vi "graph3.vi"(11 "replay":bool) -> (0 "path_size":i32, 3 "XY Graph":cluster{"Y":dbl[], "Y":dbl[]}[](graph)=[{"Y"=[-25.865695246715575, -25.865695246715575, -25.865695246715575], "Y"=[59.163033466791006, 59.163033466791006, 59.163033466791006]}, {"Y"=[0.85, 0.95, 0.95, 0.6, 0.6, 0.85, 0.85, -0.85, -0.85, -0.95, -0.95, -0.6, -0.6, -0.85, -0.6, -0.6, -0.85, -0.85, 0.85, 0.85], "Y"=[-0.6, -0.6, -1.4, -1.4, -0.6, -0.6, 2.4, 2.4, -0.6, -0.6, -1.4, -1.4, -0.6, -0.6, -0.6, -1.4, -1.4, -1.6, -1.6, -1.4]}, {"Y"=[-25.865695246715575], "Y"=[59.163033466791006]}, {"Y"=[], "Y"=[]}, {"Y"=array[926 elements], "Y"=array[926 elements]}, {"Y"=[nan, nan], "Y"=[nan, nan]}, {"Y"=[-25.865695246715575], "Y"=[59.163033466791006]}, {"Y"=[], "Y"=[]}, {"Y"=[], "Y"=[]}, {"Y"=[0.0], "Y"=[0.0]}, {"Y"=[], "Y"=[]}, {"Y"=[], "Y"=[]}, {"Y"=[691.7888277244315, 691.8377331659157, 691.8864790442867, 691.9350679862869, 691.9835025898547, 692.0317854247338, 692.079919033068, 692.1279059299806, 692.1757486041453, 692.2234495183519, 692.2710111100497, 692.3184357918904, 692.365725952261, 692.412883955801, 692.4599121439145, 692.5068128352747, 692.5535883263143, 692.6002408917145, 692.6467727848759, 692.6931862383941, 692.7394834645125, 692.785666655583, 692.8317379845035, 692.8776996051629, 692.9235536528688, 692.969302244769, 693.0149474802747, 693.060491441465, 693.1059361934975, 693.151283785001, 693.196536248471, 693.2416956006535, 693.2867638429291, 693.3317429616844, 693.3766349286853, 693.4214417014377, 693.4661652235502, 693.5108074250859, 693.5553702229134, 693.5998555210545, 693.6442652110193, 693.6886011721464, 693.7328652719325, 693.7770593663641, 693.8211853002351, 693.8652449074733, 693.9092400114525, 693.9531724253069, 693.9970439522381, 694.0408563858227, 694.0846115103164, 694.1283111009493, 694.1719569242241, 694.2155507382114, 694.259094292835, 694.3025893301664, 694.3460375847027, 694.3894407836557, 694.4328006472265, 694.476118888889, 694.5193972156585, 694.5626373283712, 694.6058409219545, 694.6490096856918, 694.6921453034947, 694.7352494541701, 694.7783238116778, 694.8213700453995, 694.8643898203949, 694.9073847976673, 694.9503566344149, 694.9933069842926, 695.0362374976652, 695.079149821865, 695.1220456014439, 695.1649264784243, 695.2077940925565, 695.2506500815632, 695.2934960813969, 695.3363337264864, 695.3791646499868, 695.4219904840265, 695.464812859962, 695.5076334086223, 695.5504537605557, 695.5932755462828, 695.6361003965429, 695.6789299425405, 695.7217658161954, 695.7646096503946, 695.807463079234, 695.8503277382761, 695.8932052647941, 695.9360972980251], "Y"=[-402.1714380892973, -402.2324443015287, -402.29325146963055, -402.3538628702814, -402.4142817442331, -402.47451129706894, -402.53455469993827, -402.5944150902866, -402.6540955725668, -402.71359921893855, -402.7729290699565, -402.832088135239, -402.8910793941361, -402.9499057963747, -403.00857026269705, -403.0670756854909, -403.12542492940014, -403.18362083193375, -403.24166620405737, -403.2995638307791, -403.3573164717253, -403.4149268617041, -403.4723977112591, -403.5297317072198, -403.58693151323575, -403.64399977030746, -403.7009390973042, -403.7577520914824, -403.81444132898264, -403.8710093653304, -403.9274587359257, -403.98379195652205, -404.0400115237071, -404.09611991536156, -404.1521195911291, -404.2080129928654, -404.2638025450895, -404.3194906554251, -404.375079715037, -404.4305720990579, -404.4859701670225, -404.5412762632748, -404.596492717394, -404.6516218445924, -404.70666594612766, -404.76162730969963, -404.81650820984265, -404.87131090831787, -404.9260376544974, -404.98069068574665, -405.0352722278018, -405.0897844951429, -405.14422969136206, -405.19861000952994, -405.2529276325616, -405.30718473357007, -405.3613834762236, -405.41552601510165, -405.46961449603776, -405.52365105647283, -405.5776378257941, -405.6315769256789, -405.685470470432, -405.7393205673213, -405.7931293169138, -405.84689881340205, -405.90063114494075, -405.9543283939694, -406.0079926375368, -406.0616259476311, -406.11523039149404, -406.1688080319476, -406.2223609277105, -406.2758911337184, -406.3294007014348, -406.38289167917463, -406.4363661124128, -406.4898260440976, -406.54327351496966, -406.5967105638653, -406.65013922803496, -406.70356154344927, -406.75697954511423, -406.8103952673769, -406.8638107442369, -406.9172280096572, -406.97064909787343, -407.0240760437018, -407.0775108828543, -407.1309556522436, -407.18441239029335, -407.23788313725817, -407.2913699355226, -407.3448748299264]}, {"Y"=[], "Y"=[]}, {"Y"=[-0.152017305614708], "Y"=[0.5451838106381299]}])   [LabVIEW 2015]
uses:
  G_NAV.vi
  G_VEH.vi
  G_SEN.vi
  G_PATH.vi
  <vilib>/Analysis/Matrix/Datatypes/RealMatrix.ctl
  <vilib>/Analysis/Matrix/NI_Matrix.lvlib
  <vilib>/Analysis/NI_AALBase.lvlib
  G_LCM.vi
  <vilib>/Analysis/baseanly.llb/Real A x B.vi
  G_ALL.vi
panel:
  out "x 17":dbl[](array[numeric])=[-13.0, -13.0, -13.0, -13.0, -13.0, -13.0, -13.0, -13.0, -13.0, -13.0, -13.0, -13.0, -13.0, -13.0, -13.0, -13.0, -13.0, -13.0, -13.0, -13.0, -13.0, -13.0, -13.0, -13.0, -13.0, -13.25, -13.25, -13.25, -13.25, -13.25, -13.25, -13.25, -13.25, -13.25, -13.25, -13.25, -13.25, -13.25, -13.25, -13.25, -13.25, -13.25, -13.25, -13.25, -13.25, -13.5, -13.25, -13.25, -13.25, -13.5, -13.5, -13.25, -13.5, -13.5, -13.5, -13.5, -13.5, -13.25, -13.5, -13.5, -13.75, -13.5, -13.5, -13.25, -13.75, -13.75, -13.5, -13.5, -13.5, -14.0, -14.0, -14.0, -13.75, -13.75, -13.75, -13.75, -1.0, -1.0, -0.75, -0.75, -0.75, -0.5, -0.5, -0.5, -0.25, -0.25, -0.25, -0.25, 0.0, 0.0, 0.0, 0.0, 0.0, 0.25, 0.25, 0.25, 0.25, 0.25, 0.5, 0.5, 0.5, 0.5, 0.75, 0.75, 0.75, 1.0, 1.0, 1.25, 1.25, 1.25, 1.5, 1.5]
  out "y 17":dbl[](array[numeric])=[0.0, 0.25, 0.5, 0.75, 1.0, 1.25, 1.25, 1.5, 1.75, 2.0, 2.25, 2.5, 2.75, 3.0, 3.25, 3.5, 3.75, 4.0, 4.25, 4.5, 4.75, 5.0, 5.25, 5.5, 5.75, 6.0, 6.5, 6.75, 7.0, 7.25, 7.5, 8.0, 8.25, 8.5, 9.0, 9.25, 9.5, 10.0, 10.25, 10.75, 11.25, 11.5, 12.0, 12.5, 13.0, 13.5, 13.75, 14.25, 14.75, 15.5, 16.0, 16.5, 17.25, 18.0, 18.5, 19.5, 20.0, 20.5, 21.75, 22.25, 23.75, 24.5, 25.25, 26.25, 28.25, 29.25, 30.5, 31.75, 33.25, 36.5, 38.25, 40.5, 42.75, 45.25, 48.25, 51.5, 4.25, 4.0, 4.0, 4.0, 3.75, 3.75, 3.75, 3.5, 3.5, 3.5, 3.25, 3.25, 3.25, 3.25, 3.25, 3.25, 3.0, 3.0, 3.0, 3.0, 3.0, 2.75, 3.0, 3.0, 3.0, 3.25, 3.25, 3.25, 3.5, 3.5, 3.5, 3.75, 3.75, 4.0, 4.0, 4.25]
  out "x 16":dbl[](array[numeric])=[-13.0, -13.0, -13.0, -13.0, -13.0, -13.0, -13.0, -13.0, -13.0, -13.0, -13.0, -13.0, -13.0, -13.0, -13.0, -13.0, -13.0, -13.0, -13.0, -13.0, -13.0, -13.0, -13.0, -13.0, -13.0, -13.25, -13.25, -13.25, -13.25, -13.25, -13.25, -13.25, -13.25, -13.25, -13.25, -13.25, -13.25, -13.25, -13.25, -13.25, -13.25, -13.25, -13.25, -13.25, -13.25, -13.5, -13.25, -13.25, -13.25, -13.5, -13.5, -13.25, -13.5, -13.5, -13.5, -13.5, -13.5, -13.25, -13.5, -13.5, -13.75, -13.5, -13.5, -13.25, -13.75, -13.75, -13.5, -13.5, -13.5, -14.0, -14.0, -14.0, -13.75, -13.75, -13.75, -13.75, -1.0, -1.0, -0.75, -0.75, -0.75, -0.5, -0.5, -0.5, -0.25, -0.25, -0.25, -0.25, 0.0, 0.0, 0.0, 0.0, 0.0, 0.25, 0.25, 0.25, 0.25, 0.25, 0.5, 0.5, 0.5, 0.5, 0.75, 0.75, 0.75, 1.0, 1.0, 1.25, 1.25, 1.25, 1.5, 1.5]
  out "y 16":dbl[](array[numeric])=[0.0, 0.25, 0.5, 0.75, 1.0, 1.25, 1.25, 1.5, 1.75, 2.0, 2.25, 2.5, 2.75, 3.0, 3.25, 3.5, 3.75, 4.0, 4.25, 4.5, 4.75, 5.0, 5.25, 5.5, 5.75, 6.0, 6.5, 6.75, 7.0, 7.25, 7.5, 8.0, 8.25, 8.5, 9.0, 9.25, 9.5, 10.0, 10.25, 10.75, 11.25, 11.5, 12.0, 12.5, 13.0, 13.5, 13.75, 14.25, 14.75, 15.5, 16.0, 16.5, 17.25, 18.0, 18.5, 19.5, 20.0, 20.5, 21.75, 22.25, 23.75, 24.5, 25.25, 26.25, 28.25, 29.25, 30.5, 31.75, 33.25, 36.5, 38.25, 40.5, 42.75, 45.25, 48.25, 51.5, 4.25, 4.0, 4.0, 4.0, 3.75, 3.75, 3.75, 3.5, 3.5, 3.5, 3.25, 3.25, 3.25, 3.25, 3.25, 3.25, 3.0, 3.0, 3.0, 3.0, 3.0, 2.75, 3.0, 3.0, 3.0, 3.25, 3.25, 3.25, 3.5, 3.5, 3.5, 3.75, 3.75, 4.0, 4.0, 4.25]
  out "M6006":T1={"GPSTime"=22892800.0, "attitude[2]"=-0.6123908, "lcc[0]"=-970.47205, "lcc[1]"=200.52362, "heading_GPS"=-0.6106907} {"GPSTime" format="%#_6f"}
  out "y 5":dbl[](array[numeric])
  out "x 5":dbl[](array[numeric])
  out "y 4":dbl[](array[numeric])
  out "x 4":dbl[](array[numeric])
  out "y 6":dbl[](array[numeric])
  out "x 6":dbl[](array[numeric])
  out "x 14":dbl[](array[numeric])
  out "y 14":dbl[](array[numeric])
  out "y 10":dbl[](array[numeric])
  out "x 10":dbl[](array[numeric])
  out "y 1":dbl[](array[numeric])
  out "x 1":dbl[](array[numeric])
  out "y 15":dbl[](array[numeric])=[0.0, 0.25, 0.5, 0.75, 1.0, 1.25, 1.25, 1.5, 1.75, 2.0, 2.25, 2.5, 2.75, 3.0, 3.25, 3.5, 3.75, 4.0, 4.25, 4.5, 4.75, 5.0, 5.25, 5.5, 5.75, 6.0, 6.5, 6.75, 7.0, 7.25, 7.5, 8.0, 8.25, 8.5, 9.0, 9.25, 9.5, 10.0, 10.25, 10.75, 11.25, 11.5, 12.0, 12.5, 13.0, 13.5, 13.75, 14.25, 14.75, 15.5, 16.0, 16.5, 17.25, 18.0, 18.5, 19.5, 20.0, 20.5, 21.75, 22.25, 23.75, 24.5, 25.25, 26.25, 28.25, 29.25, 30.5, 31.75, 33.25, 36.5, 38.25, 40.5, 42.75, 45.25, 48.25, 51.5, 4.25, 4.0, 4.0, 4.0, 3.75, 3.75, 3.75, 3.5, 3.5, 3.5, 3.25, 3.25, 3.25, 3.25, 3.25, 3.25, 3.0, 3.0, 3.0, 3.0, 3.0, 2.75, 3.0, 3.0, 3.0, 3.25, 3.25, 3.25, 3.5, 3.5, 3.5, 3.75, 3.75, 4.0, 4.0, 4.25]
  out "x 15":dbl[](array[numeric])=[-13.0, -13.0, -13.0, -13.0, -13.0, -13.0, -13.0, -13.0, -13.0, -13.0, -13.0, -13.0, -13.0, -13.0, -13.0, -13.0, -13.0, -13.0, -13.0, -13.0, -13.0, -13.0, -13.0, -13.0, -13.0, -13.25, -13.25, -13.25, -13.25, -13.25, -13.25, -13.25, -13.25, -13.25, -13.25, -13.25, -13.25, -13.25, -13.25, -13.25, -13.25, -13.25, -13.25, -13.25, -13.25, -13.5, -13.25, -13.25, -13.25, -13.5, -13.5, -13.25, -13.5, -13.5, -13.5, -13.5, -13.5, -13.25, -13.5, -13.5, -13.75, -13.5, -13.5, -13.25, -13.75, -13.75, -13.5, -13.5, -13.5, -14.0, -14.0, -14.0, -13.75, -13.75, -13.75, -13.75, -1.0, -1.0, -0.75, -0.75, -0.75, -0.5, -0.5, -0.5, -0.25, -0.25, -0.25, -0.25, 0.0, 0.0, 0.0, 0.0, 0.0, 0.25, 0.25, 0.25, 0.25, 0.25, 0.5, 0.5, 0.5, 0.5, 0.75, 0.75, 0.75, 1.0, 1.0, 1.25, 1.25, 1.25, 1.5, 1.5]
  out "y 13":dbl[](array[numeric])=[0.0, 0.25, 0.5, 0.75, 1.0, 1.25, 1.25, 1.5, 1.75, 2.0, 2.25, 2.5, 2.75, 3.0, 3.25, 3.5, 3.75, 4.0, 4.25, 4.5, 4.75, 5.0, 5.25, 5.5, 5.75, 6.0, 6.5, 6.75, 7.0, 7.25, 7.5, 8.0, 8.25, 8.5, 9.0, 9.25, 9.5, 10.0, 10.25, 10.75, 11.25, 11.5, 12.0, 12.5, 13.0, 13.5, 13.75, 14.25, 14.75, 15.5, 16.0, 16.5, 17.25, 18.0, 18.5, 19.5, 20.0, 20.5, 21.75, 22.25, 23.75, 24.5, 25.25, 26.25, 28.25, 29.25, 30.5, 31.75, 33.25, 36.5, 38.25, 40.5, 42.75, 45.25, 48.25, 51.5, 4.25, 4.0, 4.0, 4.0, 3.75, 3.75, 3.75, 3.5, 3.5, 3.5, 3.25, 3.25, 3.25, 3.25, 3.25, 3.25, 3.0, 3.0, 3.0, 3.0, 3.0, 2.75, 3.0, 3.0, 3.0, 3.25, 3.25, 3.25, 3.5, 3.5, 3.5, 3.75, 3.75, 4.0, 4.0, 4.25]
  out "x 13":dbl[](array[numeric])=[-13.0, -13.0, -13.0, -13.0, -13.0, -13.0, -13.0, -13.0, -13.0, -13.0, -13.0, -13.0, -13.0, -13.0, -13.0, -13.0, -13.0, -13.0, -13.0, -13.0, -13.0, -13.0, -13.0, -13.0, -13.0, -13.25, -13.25, -13.25, -13.25, -13.25, -13.25, -13.25, -13.25, -13.25, -13.25, -13.25, -13.25, -13.25, -13.25, -13.25, -13.25, -13.25, -13.25, -13.25, -13.25, -13.5, -13.25, -13.25, -13.25, -13.5, -13.5, -13.25, -13.5, -13.5, -13.5, -13.5, -13.5, -13.25, -13.5, -13.5, -13.75, -13.5, -13.5, -13.25, -13.75, -13.75, -13.5, -13.5, -13.5, -14.0, -14.0, -14.0, -13.75, -13.75, -13.75, -13.75, -1.0, -1.0, -0.75, -0.75, -0.75, -0.5, -0.5, -0.5, -0.25, -0.25, -0.25, -0.25, 0.0, 0.0, 0.0, 0.0, 0.0, 0.25, 0.25, 0.25, 0.25, 0.25, 0.5, 0.5, 0.5, 0.5, 0.75, 0.75, 0.75, 1.0, 1.0, 1.25, 1.25, 1.25, 1.5, 1.5]
  out "y 12":dbl[](array[numeric])=[0.0, 0.25, 0.5, 0.75, 1.0, 1.25, 1.25, 1.5, 1.75, 2.0, 2.25, 2.5, 2.75, 3.0, 3.25, 3.5, 3.75, 4.0, 4.25, 4.5, 4.75, 5.0, 5.25, 5.5, 5.75, 6.0, 6.5, 6.75, 7.0, 7.25, 7.5, 8.0, 8.25, 8.5, 9.0, 9.25, 9.5, 10.0, 10.25, 10.75, 11.25, 11.5, 12.0, 12.5, 13.0, 13.5, 13.75, 14.25, 14.75, 15.5, 16.0, 16.5, 17.25, 18.0, 18.5, 19.5, 20.0, 20.5, 21.75, 22.25, 23.75, 24.5, 25.25, 26.25, 28.25, 29.25, 30.5, 31.75, 33.25, 36.5, 38.25, 40.5, 42.75, 45.25, 48.25, 51.5, 4.25, 4.0, 4.0, 4.0, 3.75, 3.75, 3.75, 3.5, 3.5, 3.5, 3.25, 3.25, 3.25, 3.25, 3.25, 3.25, 3.0, 3.0, 3.0, 3.0, 3.0, 2.75, 3.0, 3.0, 3.0, 3.25, 3.25, 3.25, 3.5, 3.5, 3.5, 3.75, 3.75, 4.0, 4.0, 4.25]
  out "x 12":dbl[](array[numeric])=[-13.0, -13.0, -13.0, -13.0, -13.0, -13.0, -13.0, -13.0, -13.0, -13.0, -13.0, -13.0, -13.0, -13.0, -13.0, -13.0, -13.0, -13.0, -13.0, -13.0, -13.0, -13.0, -13.0, -13.0, -13.0, -13.25, -13.25, -13.25, -13.25, -13.25, -13.25, -13.25, -13.25, -13.25, -13.25, -13.25, -13.25, -13.25, -13.25, -13.25, -13.25, -13.25, -13.25, -13.25, -13.25, -13.5, -13.25, -13.25, -13.25, -13.5, -13.5, -13.25, -13.5, -13.5, -13.5, -13.5, -13.5, -13.25, -13.5, -13.5, -13.75, -13.5, -13.5, -13.25, -13.75, -13.75, -13.5, -13.5, -13.5, -14.0, -14.0, -14.0, -13.75, -13.75, -13.75, -13.75, -1.0, -1.0, -0.75, -0.75, -0.75, -0.5, -0.5, -0.5, -0.25, -0.25, -0.25, -0.25, 0.0, 0.0, 0.0, 0.0, 0.0, 0.25, 0.25, 0.25, 0.25, 0.25, 0.5, 0.5, 0.5, 0.5, 0.75, 0.75, 0.75, 1.0, 1.0, 1.25, 1.25, 1.25, 1.5, 1.5]
  out "y 11":dbl[](array[numeric])=[0.0, 0.25, 0.5, 0.75, 1.0, 1.25, 1.25, 1.5, 1.75, 2.0, 2.25, 2.5, 2.75, 3.0, 3.25, 3.5, 3.75, 4.0, 4.25, 4.5, 4.75, 5.0, 5.25, 5.5, 5.75, 6.0, 6.5, 6.75, 7.0, 7.25, 7.5, 8.0, 8.25, 8.5, 9.0, 9.25, 9.5, 10.0, 10.25, 10.75, 11.25, 11.5, 12.0, 12.5, 13.0, 13.5, 13.75, 14.25, 14.75, 15.5, 16.0, 16.5, 17.25, 18.0, 18.5, 19.5, 20.0, 20.5, 21.75, 22.25, 23.75, 24.5, 25.25, 26.25, 28.25, 29.25, 30.5, 31.75, 33.25, 36.5, 38.25, 40.5, 42.75, 45.25, 48.25, 51.5, 4.25, 4.0, 4.0, 4.0, 3.75, 3.75, 3.75, 3.5, 3.5, 3.5, 3.25, 3.25, 3.25, 3.25, 3.25, 3.25, 3.0, 3.0, 3.0, 3.0, 3.0, 2.75, 3.0, 3.0, 3.0, 3.25, 3.25, 3.25, 3.5, 3.5, 3.5, 3.75, 3.75, 4.0, 4.0, 4.25]
  out "x 11":dbl[](array[numeric])=[-13.0, -13.0, -13.0, -13.0, -13.0, -13.0, -13.0, -13.0, -13.0, -13.0, -13.0, -13.0, -13.0, -13.0, -13.0, -13.0, -13.0, -13.0, -13.0, -13.0, -13.0, -13.0, -13.0, -13.0, -13.0, -13.25, -13.25, -13.25, -13.25, -13.25, -13.25, -13.25, -13.25, -13.25, -13.25, -13.25, -13.25, -13.25, -13.25, -13.25, -13.25, -13.25, -13.25, -13.25, -13.25, -13.5, -13.25, -13.25, -13.25, -13.5, -13.5, -13.25, -13.5, -13.5, -13.5, -13.5, -13.5, -13.25, -13.5, -13.5, -13.75, -13.5, -13.5, -13.25, -13.75, -13.75, -13.5, -13.5, -13.5, -14.0, -14.0, -14.0, -13.75, -13.75, -13.75, -13.75, -1.0, -1.0, -0.75, -0.75, -0.75, -0.5, -0.5, -0.5, -0.25, -0.25, -0.25, -0.25, 0.0, 0.0, 0.0, 0.0, 0.0, 0.25, 0.25, 0.25, 0.25, 0.25, 0.5, 0.5, 0.5, 0.5, 0.75, 0.75, 0.75, 1.0, 1.0, 1.25, 1.25, 1.25, 1.5, 1.5]
  out "y 9":dbl[](array[numeric])=[-40.25486400827094, -40.04085960963455, -39.821235299880705, -39.59593792545196, -39.364914332790825, -39.12811136833988, -38.88547587854164, -38.636954709838655, -38.382494708673484, -38.12204272148863, -37.85554559472668, -37.58295017483014, -37.30420330824157, -37.0192518414035, -36.728042620758494, -36.43052249274907, -36.126638303817785, -35.81633690040717, -35.49956512895978, -35.176269835918156, -34.846397867724825, -34.50989607082233, -34.166711291653236, -33.81679037666006, -33.460080172285366, -33.09652752497168, -32.72607928116154, -32.3486822872975, -31.96428338982209, -31.57282943517787, -31.17426726980736, -30.768543740153135, -30.355605692657697, -30.338651341222633, -30.338651341222633, -29.95729378436619, -29.572397676750224, -29.183911226613308, -28.791782642194068, -28.395960131731087, -27.996391903462964, -27.593026165628288, -27.185811126465662, -26.774694994213668, -26.359625977110902, -25.940552283395995, -25.5174221213075, -25.090183699084033, -24.658785224964184, -24.22317490718656, -23.783300953989748, -23.33911157361234, -22.89055497429293, -22.43757936427013, -21.980132951782515, -21.5181639450687, -21.05162055236726, -20.58045098191681, -20.10460344195595, -19.62402614072324, -19.138667286457324, -18.648475087396758, -18.153397751780158, -17.653383487846114, -17.14838050383323, -16.6383370079801, -16.123201208525305, -15.602921313707439, -15.077445531765132, -14.546722070936944, -14.010699139461483, -13.469324945577348, -12.922547697523145, -12.370315603537431, -11.812576871858855, -11.249279710725965, -10.68037232837739, -10.105802933051706, -9.52551973298753, -8.939470936423437, -8.347604751598034, -8.312579060465806, -8.312579060465806, -7.815979397588906, -7.318560473773825, -6.820356240811432, -6.321400650492564, -5.8217276546080905, -5.321371204948849, -4.820365253305692, -4.318743751469474, -3.816540651231034, -3.313789904381253, -2.8105254627109564, -2.3067812780109964, -1.8025913020722415, -1.2979894866855162, -0.7930097836417018, -0.2876861447316371, 0.2179474782538381, 0.7238571335238572, 1.2300088692875666, 1.7363687337541345, 2.2429027751326935, 2.7495770416323975, 3.2563575814623866, 3.763210442831828, 4.270101673949855, 4.776997323025622, 5.283863438268267, 5.79066606788696, 6.297371260090832, 6.803945063089038, 7.310353525090725, 7.816562694305046, 8.322538618941149, 8.82824734720817, 9.333654927315276, 9.532792066869051, 9.532792066869058, 10.032676667529001, 10.532532309358876, 11.032359899557544, 11.53216034532386, 12.03193455385667, 12.53168343235485, 13.03140788801724, 13.531108828042706, 14.030787159630101, 14.530443789978285, 15.030079626286113, 15.529695575752449, 16.029292545576137, 16.52887144295605, 17.028433175091028, 17.527978649179936, 18.02750877242164, 18.527024452014977, 19.026526595158828, 19.526016109052026, 20.025493900893448, 20.52496087788194, 21.02441794721636, 21.523866016095567, 22.023305991718424, 22.522738781283774, 23.022165291990486, 23.521586431037413, 24.021003105623414, 24.520416222947343, 25.01982669020806, 25.51923541460442, 26.018643303335274, 26.518051263599492, 27.017460202595917, 27.51687102752342, 28.016284645580857, 28.515701963967068, 29.01512388988093, 29.51455133052128, 30.013985193087, 30.513426384776935, 31.012875812789932, 31.512334384324856, 32.01180300658057, 32.511282586755925, 33.01077403204978, 33.51027824966099, 34.00979614678842, 34.15163746485512, 34.15163746485511, 34.65085156194158, 35.150114036225105, 35.649423358614406, 36.148778000018126, 36.64817643134495, 37.14761712350358, 37.64709854740265, 38.14661917395086, 38.64617747405689, 39.14577191862942, 39.6454009785771, 40.14506312480863, 40.644756828232666, 41.14448055975791, 41.644232790293024, 42.14401199074667, 42.643816632027544, 43.14364518504432, 43.64349612070567, 44.14336790992027, 44.6432590235968, 45.14316793264393, 45.64309310797034, 46.143033020484694, 46.64298614109569, 47.14295094071199, 47.64292589024228, 48.14290946059522, 48.64290012267951, 49.142896347403784, 49.64289660567677, 50.142899368407114, 50.64290310650349, 51.14290629087459, 51.64290739242908, 52.14290488207564, 52.64289723072293, 53.142882909279656, 53.642860388654476, 54.14282813975608, 54.64278463349311, 55.14272834077427, 55.64265773250823, 56.14257127960367, 56.642467452969264, 57.142344723513695, 57.642201562145615, 58.14203643977374, 58.6418478273067, 59.141634195653204, 59.641394015721914, 60.1411257584215, 60.64082789466066, 61.14049889534806, 61.64013723139237, 62.139741373702265, 62.63930979318643, 63.138840960753534, 63.63833334731226, 64.13778542377129, 64.63719566103929, 65.1365625300249, 65.63588450163687, 66.13516004678382, 66.62661681170006, 66.62661681170006, 67.12576345342403, 67.62478981859165, 68.1236869902195, 68.62244605132406, 69.12105808492187, 69.61951417402948, 70.11780540166339, 70.61592285084015, 71.11385760457627, 71.61160074588827, 72.10914335779272, 72.6064765233061, 73.10359132544497, 73.60047884722584, 74.09713017166524, 74.59353638177971, 75.08968856058576, 75.58557779109994, 76.08119515633875, 76.57653173931875, 77.07157862305642, 77.56632689056836, 78.060767624871, 78.55489190898098, 79.04869082591473, 79.54215545868882, 80.03527689031979, 80.52804620382416, 81.02045448221844, 81.51249280851917, 82.00415226574289, 82.49542393690609, 82.98629890502534, 83.47676825311716, 83.96682306419804, 84.45645442128455, 84.9456534073932, 85.43441110554052, 85.92271859874306, 86.4105669700173, 86.89794730237979, 87.17622393756727, 87.17622393756727, 87.62090998324233, 88.06278904034333, 88.5018353078985, 88.93802298493607, 89.37132627048422, 89.80171936357122, 90.22917646322526, 90.65367176847454, 91.07517947834734, 91.49367379187183, 91.90912890807624, 92.3215190259888, 92.73081834463773, 93.13700106305124, 93.54004138025758, 93.93991349528491, 94.3365916071615, 94.73004991491554, 95.12026261757528, 95.50720391416891, 95.89084800372467, 96.27116908527078, 96.64814135783546, 97.02173902044692, 97.39193627213336, 97.75870731192305, 98.12202633884417, 98.48186755192496, 98.83820515019363, 99.19101333267841, 99.54026629840749, 99.88593824640913, 99.89953643323281, 99.89953643323281, 100.21054094201504, 100.51734678566943, 100.81989169992012, 101.11811342049135, 101.41194968310735, 101.70133822349231, 101.98621677737043, 102.26652308046596, 102.54219486850307, 102.81316987720602, 103.07938584229896, 103.34078049950615, 103.59729158455178, 103.84885683316006, 104.09541398105519, 104.33690076396141, 104.5732549176029, 104.80441417770389, 105.0303162799886, 105.2508989601812, 105.46609995400595, 105.67585699718703, 105.88010782544866, 106.07879017451506, 106.27184178011042, 106.45920037795898, 106.64080370378494, 106.81658949331246, 106.98649548226584, 107.15045940636924, 107.30841900134685, 107.46031200292295, 107.60607614682168, 107.74564916876727, 107.87896880448396, 108.00597278969595, 108.12659886012742, 108.24078475150262, 108.34846819954572, 108.44958693998096, 108.54407870853257, 108.63188124092471, 108.71293227288164, 108.78716954012754, 108.85453077838663, 108.91495372338314, 108.96837611084122, 108.97747618937277, 108.97747618937277, 109.0156550246946, 109.04983247580746, 109.08011123358501, 109.10659398890081, 109.12938343262847, 109.14858225564154, 109.16429314881364, 109.17661880301837, 109.18566190912927, 109.19152515801999, 109.19431124056405, 109.19412284763511, 109.1910626701067, 109.18523339885247, 109.17673772474595, 109.16567833866077, 109.15215793147051, 109.13627919404871, 109.11814481726906, 109.09785749200506, 109.07551990913035, 109.05123475951848, 109.02510473404305, 108.99723252357771, 108.96772081899594, 108.93667231117144, 108.90418969097772, 108.87037564928839, 108.83533287697705, 108.79916406491728, 108.7619719039827, 108.72385908504685, 108.68492829898334, 108.64528223666576, 108.60502358896771, 108.56425504676278, 108.52307930092454, 108.48159904232658, 108.4399169618425, 108.39813575034592, 108.35635809871036, 108.31468669780945, 108.27322423851678, 108.23207341170594, 108.19133690825049, 108.15111741902408, 108.11151763490025, 108.07264024675257, 108.03458794545469, 107.99746342188017, 107.96136936690259, 107.92640847139555, 107.89268342623265, 107.86029692228745, 107.82935165043357, 107.79995030154457, 107.78125898031978, 107.78125898031978, 107.75369240153198, 107.72548456275034, 107.69669916249154, 107.66739989927227, 107.63765047160923, 107.60751457801909, 107.57705591701853, 107.54633818712422, 107.51542508685286, 107.48438031472112, 107.45326756924571, 107.42215054894329, 107.39109295233057, 107.36015847792419, 107.32941082424084, 107.29891368979723, 107.26873077311004, 107.23892577269594, 107.2095623870716, 107.18070431475374, 107.15241525425903, 107.12475890410411, 107.09779896280573, 107.07159912888052, 107.04622310084521, 107.02173457721644, 106.9981972565109, 106.97567483724531, 106.95423101793631, 106.9339294971006, 106.91483397325487, 106.89700814491579, 106.88051571060006, 106.86545285263342, 106.86545285263342, 106.85123591176482, 106.8373215059327, 106.82369194296759, 106.81032953069995, 106.79721657696027, 106.78433538957903, 106.7716682763867, 106.75919754521381, 106.74690550389077, 106.73477446024813, 106.72278672211637, 106.71092459732593, 106.69917039370733, 106.68750641909104, 106.67591498130754, 106.66437838818732, 106.65287894756085, 106.64139896725864, 106.62992075511116, 106.61842661894889, 106.60689886660232, 106.59531980590192, 106.5836717446782, 106.57193699076163, 106.56009785198269, 106.54813663617186, 106.53603565115962, 106.52377720477648, 106.51134360485288, 106.49871715921937, 106.4858801757064, 106.47281496214443, 106.45950382636393, 106.44592907619545, 106.43207301946944, 106.41791796401637, 106.40344621766674, 106.38864008825105, 106.37348188359975, 106.35795391154335, 106.34203847991229, 106.32571789653713, 106.30897446924827, 106.29179050587625, 106.27414831425155, 106.2560637066309]
  out "x 9":dbl[](array[numeric])=[-22.968902627554595, -22.51700484334325, -22.067726202847595, -21.62109147813308, -21.177125441265126, -20.735852864309198, -20.297298519330727, -19.86148717839516, -19.42844361356793, -18.998192596914485, -18.57075890050028, -18.146167296390736, -17.724442556651315, -17.305609453347444, -16.889692758544577, -16.476717244308148, -16.0667076827036, -15.659688845796383, -15.255685505651932, -14.854722434335699, -14.456824403913117, -14.062016186449632, -13.67032255401068, -13.28176827866172, -12.896378132468183, -12.514176887495505, -12.135189315809143, -11.759440189474532, -11.38695428055711, -11.017756361122329, -10.651871203235629, -10.289323578962446, -9.930138260368233, -9.915595940630572, -9.915595940630572, -9.592217431479307, -9.27296664733781, -8.957904003376973, -8.64708991476769, -8.340584796680856, -8.038449064287356, -7.740743132758091, -7.447527417263952, -7.158862332975826, -6.874808295064605, -6.595425718701188, -6.320775019056462, -6.05091661130132, -5.7859109106066535, -5.525818332143363, -5.270699291082332, -5.02061420259445, -4.775623481850621, -4.535787544021732, -4.301166804278667, -4.071821677792334, -3.8478125797336116, -3.6291999252734, -3.4160441295825903, -3.2084056078320766, -3.0063447751927437, -2.809922046835485, -2.619197837931207, -2.4342325636507813, -2.255086639165114, -2.0818204796450988, -1.9144945002616136, -1.7531691161855663, -1.597904742587841, -1.4487617946393383, -1.3058006875109367, -1.1690818363735358, -1.0386656563980352, -0.9146125627553217, -0.796982970616279, -0.6858372951518088, -0.581235951532802, -0.4832393549301528, -0.3919079205147527, -0.30730206345748806, -0.22948219892925836, -0.22511372738602808, -0.22511372738602808, -0.16680067513880384, -0.11507613036628858, -0.06966705231019729, -0.03030040021222455, 0.0032968666859287954, 0.03139778914256819, 0.05427540791599236, 0.07220276376450722, 0.08545289744639678, 0.09429884971998208, 0.09901366134354672, 0.09987037307539658, 0.09714202567383796, 0.0911016598971616, 0.08202231650367428, 0.0701770362516814, 0.055838859899467026, 0.0392808282053517, 0.020775981927619973, 0.0005973618245841139, -0.020981991345463767, -0.043689036824225154, -0.06725073385338684, -0.09139404167465787, -0.11584591952973904, -0.14033332666033183, -0.164583222308123, -0.18832256571482164, -0.21127831612212852, -0.233177432771738, -0.25374687490535136, -0.27271360176467, -0.28980457259138814, -0.30474674662721396, -0.31726708311384183, -0.32147712013105156, -0.3214771201310518, -0.3322441522303675, -0.3444544578596952, -0.3580628233106866, -0.37302403487498664, -0.38929287884424707, -0.4068241415101202, -0.4255726091642576, -0.44549306809831846, -0.4665403046039335, -0.4886691049727688, -0.5118342554964762, -0.5359905424667011, -0.5610927521750875, -0.5870956709133022, -0.6139540849729826, -0.6416227806457879, -0.670056544223363, -0.6992101619973595, -0.72903842025943, -0.7594961053012258, -0.7905380034143993, -0.8221189008906022, -0.8541935840214723, -0.8867168390986828, -0.9196434524138646, -0.9529282102586762, -0.9865258989247632, -1.0203913047037911, -1.0544792138873982, -1.088744412767236, -1.1231416876349567, -1.1576258247822122, -1.192151610500654, -1.2266738310819347, -1.261147272817699, -1.2955267219995985, -1.329766964919293, -1.3638227878684193, -1.3976489771386371, -1.4312003190215978, -1.4644315998089543, -1.4972976057923506, -1.5297531232634387, -1.5617529385138709, -1.593251837835299, -1.6242046075193748, -1.6545660338577437, -1.684290903142064, -1.713334001663981, -1.7214502693093892, -1.721450269309389, -1.7494765704663608, -1.7766543195019637, -1.803010337186423, -1.8285714442899548, -1.8533644615827702, -1.8774162098350855, -1.9007535098171258, -1.9234031822991002, -1.9453920480512341, -1.966746927843737, -1.9874946424468334, -2.00766201263074, -2.027275859165667, -2.046363002821832, -2.0649502643694664, -2.083064464578773, -2.1007324242199688, -2.1179809640632783, -2.1348369048789184, -2.1513270674370997, -2.1674782725080464, -2.183317340861975, -2.198871093269103, -2.2141663504996414, -2.229229933323813, -2.244088662511829, -2.2587693588339204, -2.27329884306029, -2.2877039359611624, -2.3020114583067546, -2.316248230867277, -2.3304410744129536, -2.3446168097140014, -2.358802257540638, -2.3730242386630804, -2.387309573851546, -2.401685083876244, -2.4161775895074067, -2.430813911515237, -2.445620870669959, -2.46062528774179, -2.4758539835009468, -2.491333778717647, -2.5070914941621076, -2.523153950604546, -2.539547968815179, -2.556300369564224, -2.573437973621899, -2.5909876017584192, -2.6089760747440036, -2.6274302133488687, -2.646376838343232, -2.66584277049731, -2.68585483058132, -2.7064398393654807, -2.7276246176200143, -2.749435986115125, -2.7719007656210435, -2.7950457769079735, -2.818897840746146, -2.843483777905771, -2.8688304091570727, -2.8949645552702545, -2.921913037015548, -2.9492635082994942, -2.9492635082994942, -2.978480917327609, -3.0098270674333767, -3.043459777809386, -3.079536867648219, -3.118216156142463, -3.1596554624846984, -3.204012605867507, -3.2514454054834765, -3.3021116805251873, -3.3561692501852223, -3.4137759336561606, -3.4750895501305976, -3.5402679188011072, -3.6094688588602786, -3.682850189500691, -3.760569729914927, -3.842785299295573, -3.929654716835212, -4.021335801726423, -4.117986373161795, -4.219764250333915, -4.326827252435352, -4.439333198658707, -4.557439908196553, -4.6813052002414715, -4.811086893986051, -4.946942808622881, -5.089030763344532, -5.237508577343594, -5.392534069812648, -5.554265059944274, -5.722859366931069, -5.898474809965605, -6.081269208240471, -6.27140038094824, -6.469026147281509, -6.674304326432857, -6.88739273759486, -7.10844919996011, -7.33763153272119, -7.5750975550706805, -7.714565866361133, -7.714565866361133, -7.943178762901428, -8.177335605648189, -8.417087352842183, -8.6624849627242, -8.913579393535008, -9.170421603515402, -9.433062550906158, -9.701553193948051, -9.975944490881862, -10.256287399948372, -10.542632879388364, -10.835031887442614, -11.133535382351901, -11.438194322357017, -11.74905966569872, -12.06618237061781, -12.389613395355056, -12.719403698151243, -13.055604237247149, -13.398265970883559, -13.747439857301249, -14.10317685474099, -14.465527921443577, -14.83454401564979, -15.210276095600387, -15.592775119536174, -15.982092045697918, -16.378277832326408, -16.78138343766241, -17.19145981994672, -17.608557937420102, -18.032728748323343, -18.0496518526286, -18.0496518526286, -18.441165968034287, -18.83605201755941, -19.234360005438532, -19.636139935906236, -20.041441813197096, -20.450315641545686, -20.862811425186578, -21.278979168354343, -21.698868875283566, -22.122530550208822, -22.550014197364675, -22.98136982098571, -23.41664742530649, -23.8558970145616, -24.29916859298561, -24.746512164813097, -25.197977734278638, -25.6536153056168, -26.113474883062164, -26.5776064708493, -27.046060073212793, -27.5188856943872, -27.996133338607113, -28.4778530101071, -28.96409471312173, -29.454908451885586, -29.950344230633245, -30.450452053599268, -30.95528192501824, -31.46488384912474, -31.979307830153324, -32.49860387233859, -33.0228219799151, -33.552012157117424, -34.08622440818015, -34.625508737337846, -35.16991514882508, -35.719493646876444, -36.2742942357265, -36.83436691960981, -37.39976170276098, -37.97052858941455, -38.54671758380513, -39.12837869016727, -39.71556191273555, -40.308317255744555, -40.90669472342885, -41.01788165020217, -41.01788165020217, -41.516426075908484, -42.01529336894664, -42.514475243301945, -43.01396341295969, -43.51374959190518, -44.013825494123736, -44.514182833600636, -45.01481332432121, -45.515708680270734, -46.01686061543453, -46.51826084379791, -47.019901079346155, -47.521773036064594, -48.0238684279385, -48.526178968953204, -49.02869637309399, -49.53141235434619, -50.03431862669508, -50.53740690412599, -51.04066890062418, -51.54409633017501, -52.04768090676373, -52.55141434437569, -53.055288356996165, -53.55929465861046, -54.0634249632039, -54.56767098476177, -55.072024437269384, -55.576477034712035, -56.08102049107504, -56.58564652034369, -57.090346836503294, -57.59511315353915, -58.09993718543659, -58.60481064618088, -59.109725249757346, -59.61467271015128, -60.119644741348004, -60.62463305733281, -61.129629372090996, -61.63462539960787, -62.13961285386874, -62.64458344885892, -63.149528898563695, -63.65444091696837, -64.15931121805825, -64.66413151581865, -65.16889352423487, -65.67358895729222, -66.17820952897598, -66.68274695327148, -67.18719294416401, -67.69153921563887, -68.19577748168139, -68.69989945627682, -69.20389685341053, -69.53980106644636, -69.53980106644636, -70.03904068922449, -70.53824534388608, -71.03741850393202, -71.53656364286319, -72.03568423418045, -72.53478375138471, -73.03386566797683, -73.53293345745773, -74.03199059332825, -74.5310405490893, -75.03008679824175, -75.52913281428651, -76.02818207072443, -76.5272380410564, -77.02630419878331, -77.52538401740605, -78.02448097042549, -78.52359853134253, -79.02274017365804, -79.52190937087288, -80.02110959648799, -80.5203443240042, -81.01961702692243, -81.51893117874353, -82.01829025296841, -82.51769772309794, -83.01715706263303, -83.51667174507452, -84.01624524392331, -84.5158810326803, -85.01558258484634, -85.51535337392235, -86.0151968734092, -86.51398695208124, -86.51398695208124, -87.01378481453521, -87.51359137792667, -88.01340613342705, -88.51322857220782, -89.01305818544041, -89.51289446429632, -90.01273689994701, -90.51258498356393, -91.01243820631852, -91.5122960593823, -92.01215803392664, -92.51202362112309, -93.01189231214308, -93.51176359815807, -94.01163697033948, -94.51151191985885, -95.01138793788758, -95.51126451559716, -96.01114114415904, -96.51101731474469, -97.01089251852558, -97.51076624667314, -98.01063799035886, -98.5105072407542, -99.01037348903058, -99.51023622635952, -100.01009494391245, -100.50994913286084, -101.00979828437613, -101.50964188962982, -102.00947943979334, -102.50931042603817, -103.00913433953575, -103.50895067145754, -104.00875891297504, -104.50855855525968, -105.00834908948293, -105.50813000681626, -106.0079007984311, -106.50766095549893, -107.00740996919122, -107.50714733067944, -108.00687253113502, -108.50658506172944, -109.00628441363415, -109.50505830995377]
  out "x 7":dbl[](array[numeric])=[0.0, -0.062285707493046516, -0.2310475110116812]
  out "y 7":dbl[](array[numeric])=[0.0, 3.113870125529085, 5.994064450521981]
  out "y 8":dbl[](array[numeric])=[-40.25486400827094, -40.04085960963455, -39.821235299880705, -39.59593792545196, -39.364914332790825, -39.12811136833988, -38.88547587854164, -38.636954709838655, -38.382494708673484, -38.12204272148863, -37.85554559472668, -37.58295017483014, -37.30420330824157, -37.0192518414035, -36.728042620758494, -36.43052249274907, -36.126638303817785, -35.81633690040717, -35.49956512895978, -35.176269835918156, -34.846397867724825, -34.50989607082233, -34.166711291653236, -33.81679037666006, -33.460080172285366, -33.09652752497168, -32.72607928116154, -32.3486822872975, -31.96428338982209, -31.57282943517787, -31.17426726980736, -30.768543740153135, -30.355605692657697, -30.338651341222633, -30.338651341222633, -29.95729378436619, -29.572397676750224, -29.183911226613308, -28.791782642194068, -28.395960131731087, -27.996391903462964, -27.593026165628288, -27.185811126465662, -26.774694994213668, -26.359625977110902, -25.940552283395995, -25.5174221213075, -25.090183699084033, -24.658785224964184, -24.22317490718656, -23.783300953989748, -23.33911157361234, -22.89055497429293, -22.43757936427013, -21.980132951782515, -21.5181639450687, -21.05162055236726, -20.58045098191681, -20.10460344195595, -19.62402614072324, -19.138667286457324, -18.648475087396758, -18.153397751780158, -17.653383487846114, -17.14838050383323, -16.6383370079801, -16.123201208525305, -15.602921313707439, -15.077445531765132, -14.546722070936944, -14.010699139461483, -13.469324945577348, -12.922547697523145, -12.370315603537431, -11.812576871858855, -11.249279710725965, -10.68037232837739, -10.105802933051706, -9.52551973298753, -8.939470936423437, -8.347604751598034, -8.312579060465806, -8.312579060465806, -7.815979397588906, -7.318560473773825, -6.820356240811432, -6.321400650492564, -5.8217276546080905, -5.321371204948849, -4.820365253305692, -4.318743751469474, -3.816540651231034, -3.313789904381253, -2.8105254627109564, -2.3067812780109964, -1.8025913020722415, -1.2979894866855162, -0.7930097836417018, -0.2876861447316371, 0.2179474782538381, 0.7238571335238572, 1.2300088692875666, 1.7363687337541345, 2.2429027751326935, 2.7495770416323975, 3.2563575814623866, 3.763210442831828, 4.270101673949855, 4.776997323025622, 5.283863438268267, 5.79066606788696, 6.297371260090832, 6.803945063089038, 7.310353525090725, 7.816562694305046, 8.322538618941149, 8.82824734720817, 9.333654927315276, 9.532792066869051, 9.532792066869058, 10.032676667529001, 10.532532309358876, 11.032359899557544, 11.53216034532386, 12.03193455385667, 12.53168343235485, 13.03140788801724, 13.531108828042706, 14.030787159630101, 14.530443789978285, 15.030079626286113, 15.529695575752449, 16.029292545576137, 16.52887144295605, 17.028433175091028, 17.527978649179936, 18.02750877242164, 18.527024452014977, 19.026526595158828, 19.526016109052026, 20.025493900893448, 20.52496087788194, 21.02441794721636, 21.523866016095567, 22.023305991718424, 22.522738781283774, 23.022165291990486, 23.521586431037413, 24.021003105623414, 24.520416222947343, 25.01982669020806, 25.51923541460442, 26.018643303335274, 26.518051263599492, 27.017460202595917, 27.51687102752342, 28.016284645580857, 28.515701963967068, 29.01512388988093, 29.51455133052128, 30.013985193087, 30.513426384776935, 31.012875812789932, 31.512334384324856, 32.01180300658057, 32.511282586755925, 33.01077403204978, 33.51027824966099, 34.00979614678842, 34.15163746485512, 34.15163746485511, 34.65085156194158, 35.150114036225105, 35.649423358614406, 36.148778000018126, 36.64817643134495, 37.14761712350358, 37.64709854740265, 38.14661917395086, 38.64617747405689, 39.14577191862942, 39.6454009785771, 40.14506312480863, 40.644756828232666, 41.14448055975791, 41.644232790293024, 42.14401199074667, 42.643816632027544, 43.14364518504432, 43.64349612070567, 44.14336790992027, 44.6432590235968, 45.14316793264393, 45.64309310797034, 46.143033020484694, 46.64298614109569, 47.14295094071199, 47.64292589024228, 48.14290946059522, 48.64290012267951, 49.142896347403784, 49.64289660567677, 50.142899368407114, 50.64290310650349, 51.14290629087459, 51.64290739242908, 52.14290488207564, 52.64289723072293, 53.142882909279656, 53.642860388654476, 54.14282813975608, 54.64278463349311, 55.14272834077427, 55.64265773250823, 56.14257127960367, 56.642467452969264, 57.142344723513695, 57.642201562145615, 58.14203643977374, 58.6418478273067, 59.141634195653204, 59.641394015721914, 60.1411257584215, 60.64082789466066, 61.14049889534806, 61.64013723139237, 62.139741373702265, 62.63930979318643, 63.138840960753534, 63.63833334731226, 64.13778542377129, 64.63719566103929, 65.1365625300249, 65.63588450163687, 66.13516004678382, 66.62661681170006, 66.62661681170006, 67.12576345342403, 67.62478981859165, 68.1236869902195, 68.62244605132406, 69.12105808492187, 69.61951417402948, 70.11780540166339, 70.61592285084015, 71.11385760457627, 71.61160074588827, 72.10914335779272, 72.6064765233061, 73.10359132544497, 73.60047884722584, 74.09713017166524, 74.59353638177971, 75.08968856058576, 75.58557779109994, 76.08119515633875, 76.57653173931875, 77.07157862305642, 77.56632689056836, 78.060767624871, 78.55489190898098, 79.04869082591473, 79.54215545868882, 80.03527689031979, 80.52804620382416, 81.02045448221844, 81.51249280851917, 82.00415226574289, 82.49542393690609, 82.98629890502534, 83.47676825311716, 83.96682306419804, 84.45645442128455, 84.9456534073932, 85.43441110554052, 85.92271859874306, 86.4105669700173, 86.89794730237979, 87.17622393756727, 87.17622393756727, 87.62090998324233, 88.06278904034333, 88.5018353078985, 88.93802298493607, 89.37132627048422, 89.80171936357122, 90.22917646322526, 90.65367176847454, 91.07517947834734, 91.49367379187183, 91.90912890807624, 92.3215190259888, 92.73081834463773, 93.13700106305124, 93.54004138025758, 93.93991349528491, 94.3365916071615, 94.73004991491554, 95.12026261757528, 95.50720391416891, 95.89084800372467, 96.27116908527078, 96.64814135783546, 97.02173902044692, 97.39193627213336, 97.75870731192305, 98.12202633884417, 98.48186755192496, 98.83820515019363, 99.19101333267841, 99.54026629840749, 99.88593824640913, 99.89953643323281, 99.89953643323281, 100.21054094201504, 100.51734678566943, 100.81989169992012, 101.11811342049135, 101.41194968310735, 101.70133822349231, 101.98621677737043, 102.26652308046596, 102.54219486850307, 102.81316987720602, 103.07938584229896, 103.34078049950615, 103.59729158455178, 103.84885683316006, 104.09541398105519, 104.33690076396141, 104.5732549176029, 104.80441417770389, 105.0303162799886, 105.2508989601812, 105.46609995400595, 105.67585699718703, 105.88010782544866, 106.07879017451506, 106.27184178011042, 106.45920037795898, 106.64080370378494, 106.81658949331246, 106.98649548226584, 107.15045940636924, 107.30841900134685, 107.46031200292295, 107.60607614682168, 107.74564916876727, 107.87896880448396, 108.00597278969595, 108.12659886012742, 108.24078475150262, 108.34846819954572, 108.44958693998096, 108.54407870853257, 108.63188124092471, 108.71293227288164, 108.78716954012754, 108.85453077838663, 108.91495372338314, 108.96837611084122, 108.97747618937277, 108.97747618937277, 109.0156550246946, 109.04983247580746, 109.08011123358501, 109.10659398890081, 109.12938343262847, 109.14858225564154, 109.16429314881364, 109.17661880301837, 109.18566190912927, 109.19152515801999, 109.19431124056405, 109.19412284763511, 109.1910626701067, 109.18523339885247, 109.17673772474595, 109.16567833866077, 109.15215793147051, 109.13627919404871, 109.11814481726906, 109.09785749200506, 109.07551990913035, 109.05123475951848, 109.02510473404305, 108.99723252357771, 108.96772081899594, 108.93667231117144, 108.90418969097772, 108.87037564928839, 108.83533287697705, 108.79916406491728, 108.7619719039827, 108.72385908504685, 108.68492829898334, 108.64528223666576, 108.60502358896771, 108.56425504676278, 108.52307930092454, 108.48159904232658, 108.4399169618425, 108.39813575034592, 108.35635809871036, 108.31468669780945, 108.27322423851678, 108.23207341170594, 108.19133690825049, 108.15111741902408, 108.11151763490025, 108.07264024675257, 108.03458794545469, 107.99746342188017, 107.96136936690259, 107.92640847139555, 107.89268342623265, 107.86029692228745, 107.82935165043357, 107.79995030154457, 107.78125898031978, 107.78125898031978, 107.75369240153198, 107.72548456275034, 107.69669916249154, 107.66739989927227, 107.63765047160923, 107.60751457801909, 107.57705591701853, 107.54633818712422, 107.51542508685286, 107.48438031472112, 107.45326756924571, 107.42215054894329, 107.39109295233057, 107.36015847792419, 107.32941082424084, 107.29891368979723, 107.26873077311004, 107.23892577269594, 107.2095623870716, 107.18070431475374, 107.15241525425903, 107.12475890410411, 107.09779896280573, 107.07159912888052, 107.04622310084521, 107.02173457721644, 106.9981972565109, 106.97567483724531, 106.95423101793631, 106.9339294971006, 106.91483397325487, 106.89700814491579, 106.88051571060006, 106.86545285263342, 106.86545285263342, 106.85123591176482, 106.8373215059327, 106.82369194296759, 106.81032953069995, 106.79721657696027, 106.78433538957903, 106.7716682763867, 106.75919754521381, 106.74690550389077, 106.73477446024813, 106.72278672211637, 106.71092459732593, 106.69917039370733, 106.68750641909104, 106.67591498130754, 106.66437838818732, 106.65287894756085, 106.64139896725864, 106.62992075511116, 106.61842661894889, 106.60689886660232, 106.59531980590192, 106.5836717446782, 106.57193699076163, 106.56009785198269, 106.54813663617186, 106.53603565115962, 106.52377720477648, 106.51134360485288, 106.49871715921937, 106.4858801757064, 106.47281496214443, 106.45950382636393, 106.44592907619545, 106.43207301946944, 106.41791796401637, 106.40344621766674, 106.38864008825105, 106.37348188359975, 106.35795391154335, 106.34203847991229, 106.32571789653713, 106.30897446924827, 106.29179050587625, 106.27414831425155, 106.2560637066309]
  out "x 8":dbl[](array[numeric])=[-22.968902627554595, -22.51700484334325, -22.067726202847595, -21.62109147813308, -21.177125441265126, -20.735852864309198, -20.297298519330727, -19.86148717839516, -19.42844361356793, -18.998192596914485, -18.57075890050028, -18.146167296390736, -17.724442556651315, -17.305609453347444, -16.889692758544577, -16.476717244308148, -16.0667076827036, -15.659688845796383, -15.255685505651932, -14.854722434335699, -14.456824403913117, -14.062016186449632, -13.67032255401068, -13.28176827866172, -12.896378132468183, -12.514176887495505, -12.135189315809143, -11.759440189474532, -11.38695428055711, -11.017756361122329, -10.651871203235629, -10.289323578962446, -9.930138260368233, -9.915595940630572, -9.915595940630572, -9.592217431479307, -9.27296664733781, -8.957904003376973, -8.64708991476769, -8.340584796680856, -8.038449064287356, -7.740743132758091, -7.447527417263952, -7.158862332975826, -6.874808295064605, -6.595425718701188, -6.320775019056462, -6.05091661130132, -5.7859109106066535, -5.525818332143363, -5.270699291082332, -5.02061420259445, -4.775623481850621, -4.535787544021732, -4.301166804278667, -4.071821677792334, -3.8478125797336116, -3.6291999252734, -3.4160441295825903, -3.2084056078320766, -3.0063447751927437, -2.809922046835485, -2.619197837931207, -2.4342325636507813, -2.255086639165114, -2.0818204796450988, -1.9144945002616136, -1.7531691161855663, -1.597904742587841, -1.4487617946393383, -1.3058006875109367, -1.1690818363735358, -1.0386656563980352, -0.9146125627553217, -0.796982970616279, -0.6858372951518088, -0.581235951532802, -0.4832393549301528, -0.3919079205147527, -0.30730206345748806, -0.22948219892925836, -0.22511372738602808, -0.22511372738602808, -0.16680067513880384, -0.11507613036628858, -0.06966705231019729, -0.03030040021222455, 0.0032968666859287954, 0.03139778914256819, 0.05427540791599236, 0.07220276376450722, 0.08545289744639678, 0.09429884971998208, 0.09901366134354672, 0.09987037307539658, 0.09714202567383796, 0.0911016598971616, 0.08202231650367428, 0.0701770362516814, 0.055838859899467026, 0.0392808282053517, 0.020775981927619973, 0.0005973618245841139, -0.020981991345463767, -0.043689036824225154, -0.06725073385338684, -0.09139404167465787, -0.11584591952973904, -0.14033332666033183, -0.164583222308123, -0.18832256571482164, -0.21127831612212852, -0.233177432771738, -0.25374687490535136, -0.27271360176467, -0.28980457259138814, -0.30474674662721396, -0.31726708311384183, -0.32147712013105156, -0.3214771201310518, -0.3322441522303675, -0.3444544578596952, -0.3580628233106866, -0.37302403487498664, -0.38929287884424707, -0.4068241415101202, -0.4255726091642576, -0.44549306809831846, -0.4665403046039335, -0.4886691049727688, -0.5118342554964762, -0.5359905424667011, -0.5610927521750875, -0.5870956709133022, -0.6139540849729826, -0.6416227806457879, -0.670056544223363, -0.6992101619973595, -0.72903842025943, -0.7594961053012258, -0.7905380034143993, -0.8221189008906022, -0.8541935840214723, -0.8867168390986828, -0.9196434524138646, -0.9529282102586762, -0.9865258989247632, -1.0203913047037911, -1.0544792138873982, -1.088744412767236, -1.1231416876349567, -1.1576258247822122, -1.192151610500654, -1.2266738310819347, -1.261147272817699, -1.2955267219995985, -1.329766964919293, -1.3638227878684193, -1.3976489771386371, -1.4312003190215978, -1.4644315998089543, -1.4972976057923506, -1.5297531232634387, -1.5617529385138709, -1.593251837835299, -1.6242046075193748, -1.6545660338577437, -1.684290903142064, -1.713334001663981, -1.7214502693093892, -1.721450269309389, -1.7494765704663608, -1.7766543195019637, -1.803010337186423, -1.8285714442899548, -1.8533644615827702, -1.8774162098350855, -1.9007535098171258, -1.9234031822991002, -1.9453920480512341, -1.966746927843737, -1.9874946424468334, -2.00766201263074, -2.027275859165667, -2.046363002821832, -2.0649502643694664, -2.083064464578773, -2.1007324242199688, -2.1179809640632783, -2.1348369048789184, -2.1513270674370997, -2.1674782725080464, -2.183317340861975, -2.198871093269103, -2.2141663504996414, -2.229229933323813, -2.244088662511829, -2.2587693588339204, -2.27329884306029, -2.2877039359611624, -2.3020114583067546, -2.316248230867277, -2.3304410744129536, -2.3446168097140014, -2.358802257540638, -2.3730242386630804, -2.387309573851546, -2.401685083876244, -2.4161775895074067, -2.430813911515237, -2.445620870669959, -2.46062528774179, -2.4758539835009468, -2.491333778717647, -2.5070914941621076, -2.523153950604546, -2.539547968815179, -2.556300369564224, -2.573437973621899, -2.5909876017584192, -2.6089760747440036, -2.6274302133488687, -2.646376838343232, -2.66584277049731, -2.68585483058132, -2.7064398393654807, -2.7276246176200143, -2.749435986115125, -2.7719007656210435, -2.7950457769079735, -2.818897840746146, -2.843483777905771, -2.8688304091570727, -2.8949645552702545, -2.921913037015548, -2.9492635082994942, -2.9492635082994942, -2.978480917327609, -3.0098270674333767, -3.043459777809386, -3.079536867648219, -3.118216156142463, -3.1596554624846984, -3.204012605867507, -3.2514454054834765, -3.3021116805251873, -3.3561692501852223, -3.4137759336561606, -3.4750895501305976, -3.5402679188011072, -3.6094688588602786, -3.682850189500691, -3.760569729914927, -3.842785299295573, -3.929654716835212, -4.021335801726423, -4.117986373161795, -4.219764250333915, -4.326827252435352, -4.439333198658707, -4.557439908196553, -4.6813052002414715, -4.811086893986051, -4.946942808622881, -5.089030763344532, -5.237508577343594, -5.392534069812648, -5.554265059944274, -5.722859366931069, -5.898474809965605, -6.081269208240471, -6.27140038094824, -6.469026147281509, -6.674304326432857, -6.88739273759486, -7.10844919996011, -7.33763153272119, -7.5750975550706805, -7.714565866361133, -7.714565866361133, -7.943178762901428, -8.177335605648189, -8.417087352842183, -8.6624849627242, -8.913579393535008, -9.170421603515402, -9.433062550906158, -9.701553193948051, -9.975944490881862, -10.256287399948372, -10.542632879388364, -10.835031887442614, -11.133535382351901, -11.438194322357017, -11.74905966569872, -12.06618237061781, -12.389613395355056, -12.719403698151243, -13.055604237247149, -13.398265970883559, -13.747439857301249, -14.10317685474099, -14.465527921443577, -14.83454401564979, -15.210276095600387, -15.592775119536174, -15.982092045697918, -16.378277832326408, -16.78138343766241, -17.19145981994672, -17.608557937420102, -18.032728748323343, -18.0496518526286, -18.0496518526286, -18.441165968034287, -18.83605201755941, -19.234360005438532, -19.636139935906236, -20.041441813197096, -20.450315641545686, -20.862811425186578, -21.278979168354343, -21.698868875283566, -22.122530550208822, -22.550014197364675, -22.98136982098571, -23.41664742530649, -23.8558970145616, -24.29916859298561, -24.746512164813097, -25.197977734278638, -25.6536153056168, -26.113474883062164, -26.5776064708493, -27.046060073212793, -27.5188856943872, -27.996133338607113, -28.4778530101071, -28.96409471312173, -29.454908451885586, -29.950344230633245, -30.450452053599268, -30.95528192501824, -31.46488384912474, -31.979307830153324, -32.49860387233859, -33.0228219799151, -33.552012157117424, -34.08622440818015, -34.625508737337846, -35.16991514882508, -35.719493646876444, -36.2742942357265, -36.83436691960981, -37.39976170276098, -37.97052858941455, -38.54671758380513, -39.12837869016727, -39.71556191273555, -40.308317255744555, -40.90669472342885, -41.01788165020217, -41.01788165020217, -41.516426075908484, -42.01529336894664, -42.514475243301945, -43.01396341295969, -43.51374959190518, -44.013825494123736, -44.514182833600636, -45.01481332432121, -45.515708680270734, -46.01686061543453, -46.51826084379791, -47.019901079346155, -47.521773036064594, -48.0238684279385, -48.526178968953204, -49.02869637309399, -49.53141235434619, -50.03431862669508, -50.53740690412599, -51.04066890062418, -51.54409633017501, -52.04768090676373, -52.55141434437569, -53.055288356996165, -53.55929465861046, -54.0634249632039, -54.56767098476177, -55.072024437269384, -55.576477034712035, -56.08102049107504, -56.58564652034369, -57.090346836503294, -57.59511315353915, -58.09993718543659, -58.60481064618088, -59.109725249757346, -59.61467271015128, -60.119644741348004, -60.62463305733281, -61.129629372090996, -61.63462539960787, -62.13961285386874, -62.64458344885892, -63.149528898563695, -63.65444091696837, -64.15931121805825, -64.66413151581865, -65.16889352423487, -65.67358895729222, -66.17820952897598, -66.68274695327148, -67.18719294416401, -67.69153921563887, -68.19577748168139, -68.69989945627682, -69.20389685341053, -69.53980106644636, -69.53980106644636, -70.03904068922449, -70.53824534388608, -71.03741850393202, -71.53656364286319, -72.03568423418045, -72.53478375138471, -73.03386566797683, -73.53293345745773, -74.03199059332825, -74.5310405490893, -75.03008679824175, -75.52913281428651, -76.02818207072443, -76.5272380410564, -77.02630419878331, -77.52538401740605, -78.02448097042549, -78.52359853134253, -79.02274017365804, -79.52190937087288, -80.02110959648799, -80.5203443240042, -81.01961702692243, -81.51893117874353, -82.01829025296841, -82.51769772309794, -83.01715706263303, -83.51667174507452, -84.01624524392331, -84.5158810326803, -85.01558258484634, -85.51535337392235, -86.0151968734092, -86.51398695208124, -86.51398695208124, -87.01378481453521, -87.51359137792667, -88.01340613342705, -88.51322857220782, -89.01305818544041, -89.51289446429632, -90.01273689994701, -90.51258498356393, -91.01243820631852, -91.5122960593823, -92.01215803392664, -92.51202362112309, -93.01189231214308, -93.51176359815807, -94.01163697033948, -94.51151191985885, -95.01138793788758, -95.51126451559716, -96.01114114415904, -96.51101731474469, -97.01089251852558, -97.51076624667314, -98.01063799035886, -98.5105072407542, -99.01037348903058, -99.51023622635952, -100.01009494391245, -100.50994913286084, -101.00979828437613, -101.50964188962982, -102.00947943979334, -102.50931042603817, -103.00913433953575, -103.50895067145754, -104.00875891297504, -104.50855855525968, -105.00834908948293, -105.50813000681626, -106.0079007984311, -106.50766095549893, -107.00740996919122, -107.50714733067944, -108.00687253113502, -108.50658506172944, -109.00628441363415, -109.50505830995377]
  out "y 3":dbl[](array[numeric])
  out "x 3":dbl[](array[numeric])
  out "y 2":dbl[](array[numeric])
  out "x 2":dbl[](array[numeric])
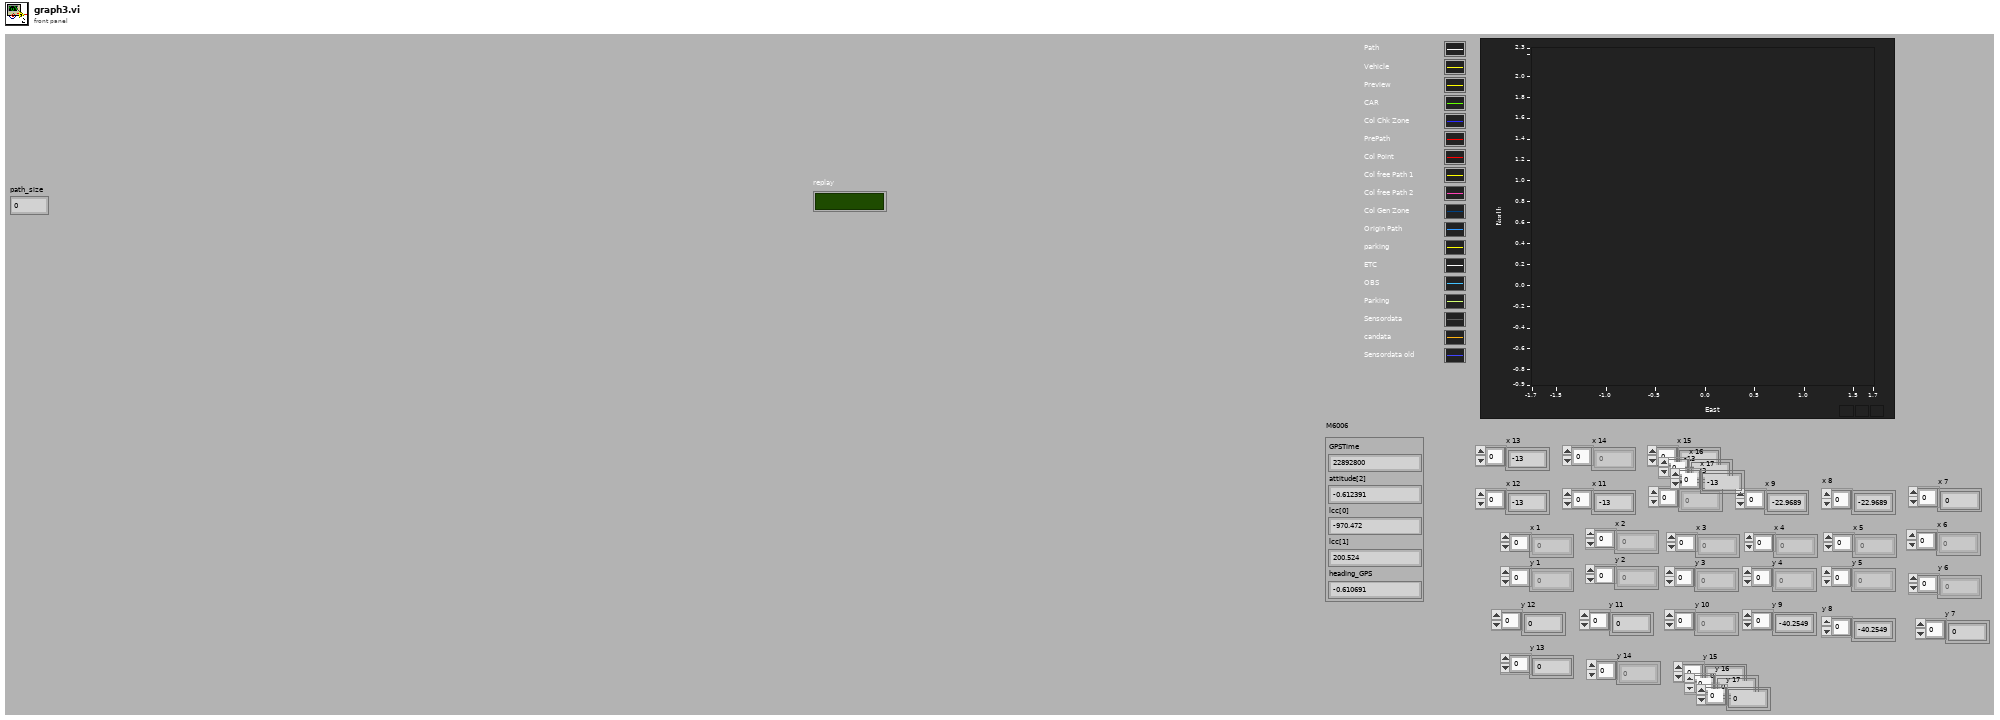
[diagram p1: front panel]
types:
  T1 = cluster{"GPSTime":dbl, "attitude[2]":sgl, "lcc[0]":sgl, "lcc[1]":sgl, "heading_GPS":sgl}
  T2 = typedef "NI_Matrix.lvlib/RealMatrix.ctl" = dbl[][]
  T3 = cluster{"Steer_input":dbl, "Steer_output":dbl, "VS_des":dbl, "VS_can":dbl, "heading":dbl, "auto":bool, "run":bool, "x":dbl, "y":dbl}
  T4 = cluster{"idx":i32, "x":dbl, "y":dbl, "h":dbl, "x_path":dbl}
  T5 = cluster{"idx":i32, "x":dbl, "y":dbl, "hp":dbl, "x_path":dbl}[]
  T6 = cluster{"hash":i64, "sys time":i64, "Auto":bool, "Run":bool, "Solenoid":bool, "T lim":bool, "brk_enc":u8, "B PWM":u16, "T PWM":u16, "ref_vel":dbl, "ref_bkr_enc":dbl, "ref_apv":dbl, "ref_steer":dbl}
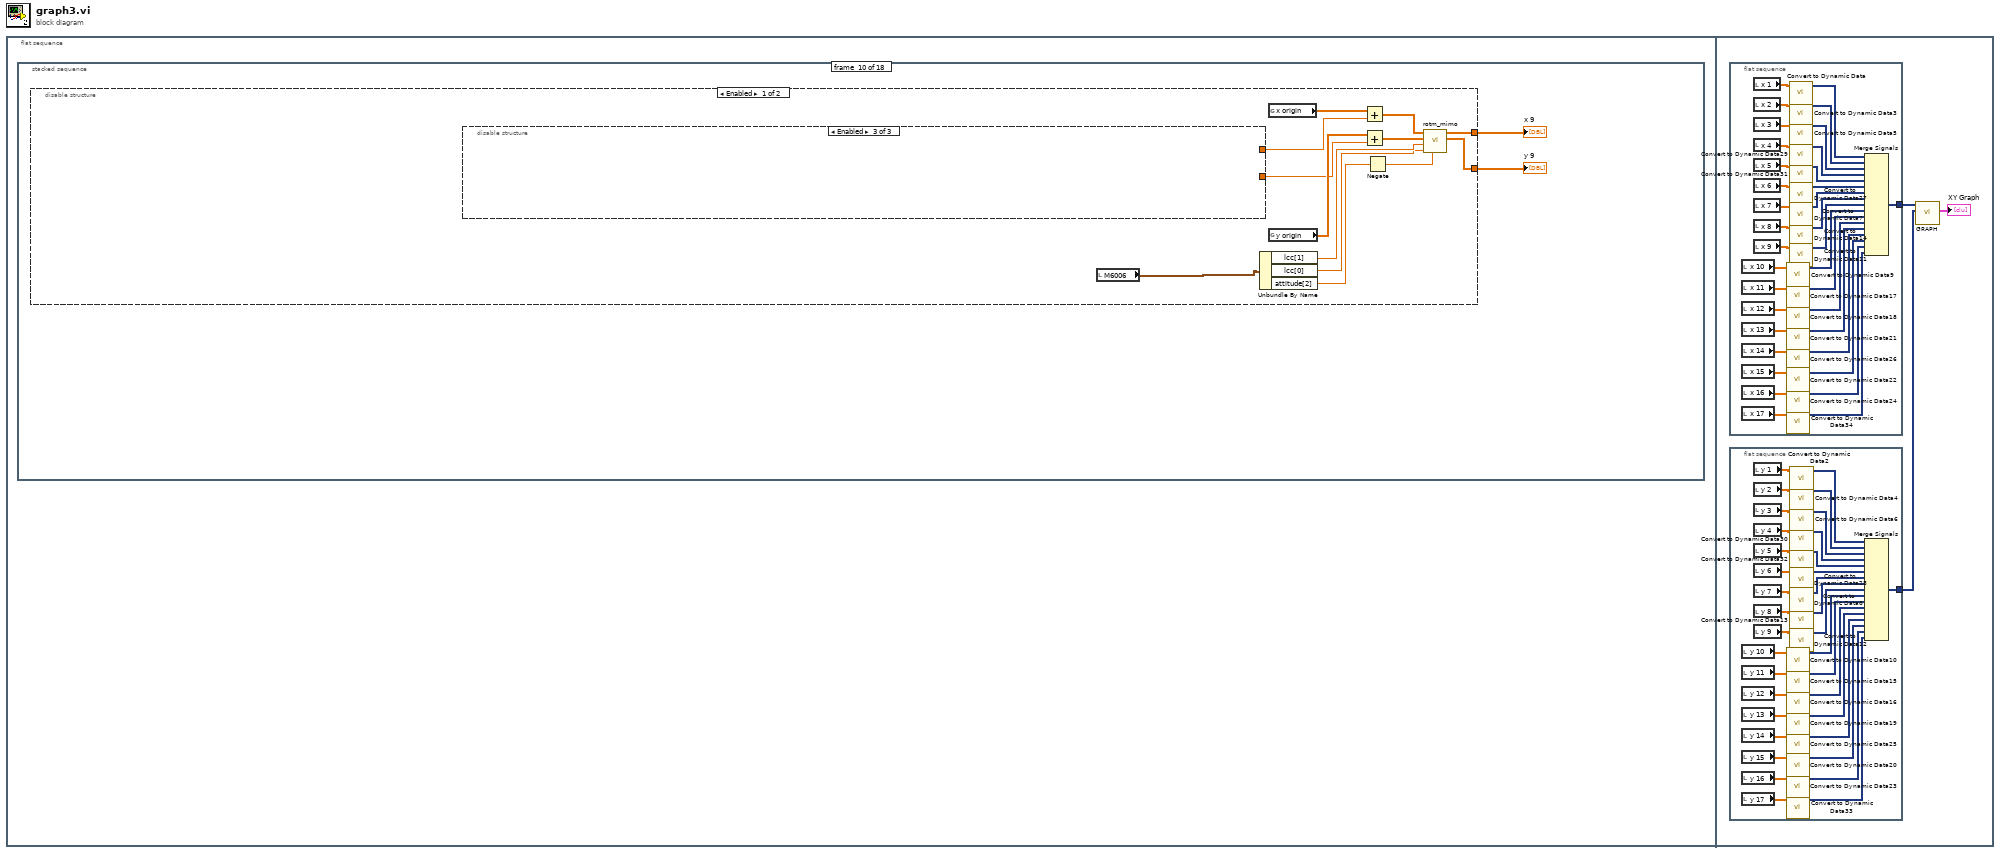
[diagram p0: block diagram]
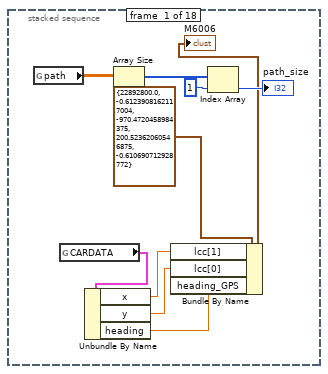
[diagram p2: hidden frame]
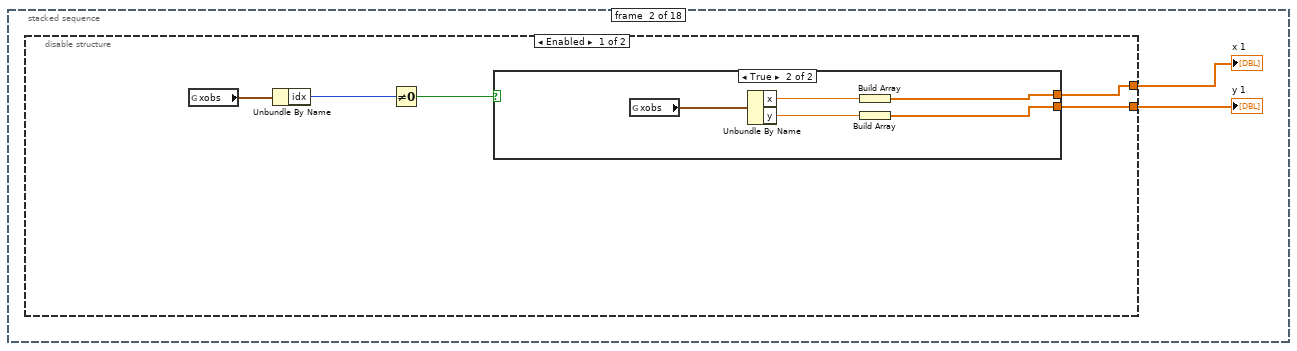
[diagram p3: hidden frame]
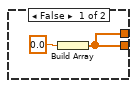
[diagram p4: hidden frame]
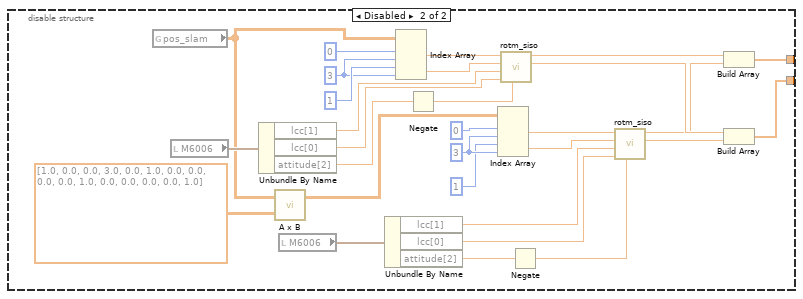
[diagram p5: hidden frame]
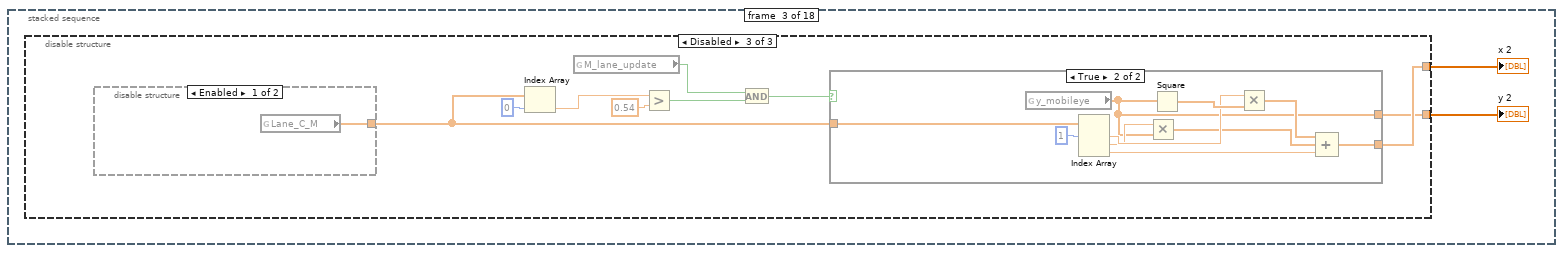
[diagram p6: hidden frame]
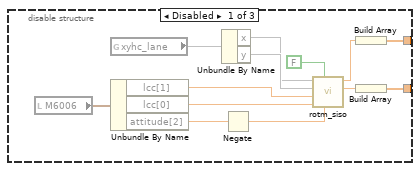
[diagram p7: hidden frame]
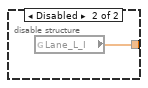
[diagram p9: hidden frame]
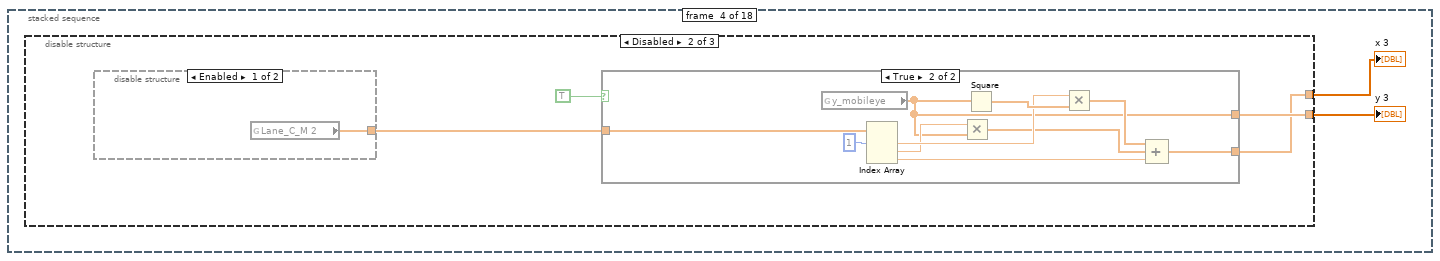
[diagram p11: hidden frame]
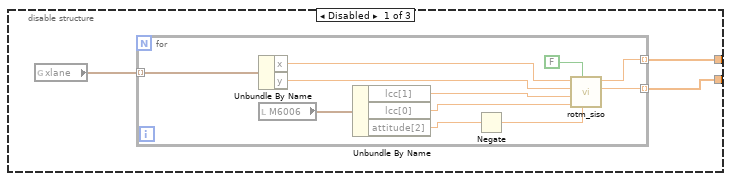
[diagram p12: hidden frame]
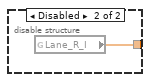
[diagram p13: hidden frame]
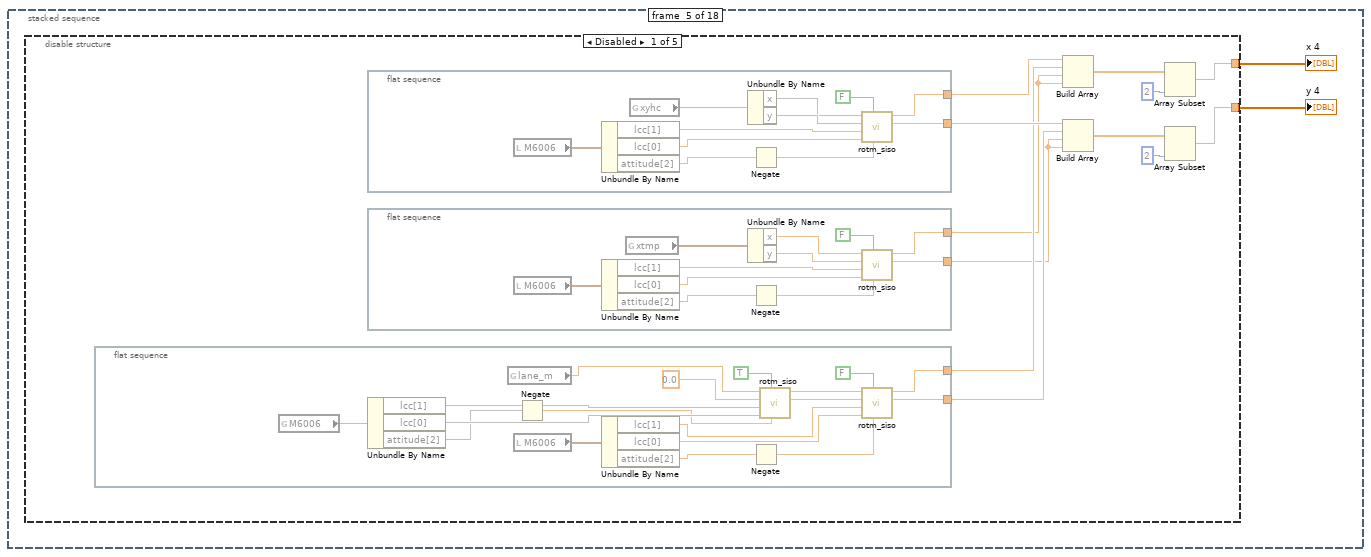
[diagram p16: hidden frame]
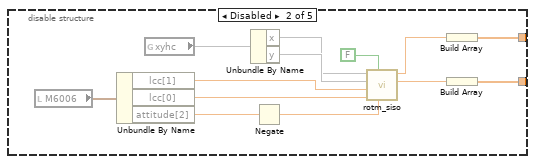
[diagram p17: hidden frame]
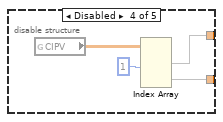
[diagram p19: hidden frame]
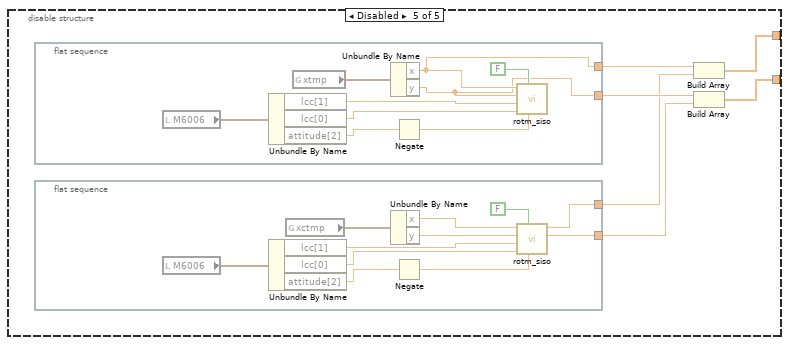
[diagram p20: hidden frame]
diagram:
  n1 = flat-sequence {
    frame #0 {
      n2 = stacked-sequence {
        frame #0 {
          n3 = global read "G_PATH.vi" "path"() -> (w7:dbl[][])
          n4 = global read "G_ALL.vi" "CARDATA"() -> (w4:T3)
          n5 = Unbundle By Name(w4) -> ("x"=w3:dbl, "y"=w2:dbl, "heading"=w1:dbl)
          n6 = Array Size(array=w7) -> (size(s)=w10:i32[])
          n7 = Bundle By Name(cluster=T1 {"GPSTime"=22892800.0, "attitude[2]"=-0.6123908, "lcc[0]"=-970.47205, "lcc[1]"=200.52362, "heading_GPS"=-0.6106907} ("M6006"), "lcc[1]"=w3, "lcc[0]"=w2, "heading_GPS"=w1) -> (→"M6006":T1)
          n8 = Index Array(array=w10, index=1) -> (element=→"path_size":i32)
        }
        frame #1 {
          n9 = disable-structure shown="Enabled" {
            disable-tunnel: [w14 w50] -> w12
            disable-tunnel: [w13 w49] -> w11
            frame Enabled {
              n10 = global read "G_VEH.vi" "xobs"() -> (w17:T4)
              n11 = Unbundle By Name(w17) -> ("idx"=w16:i32)
              n12 = Not Equal To 0?(x=w16) -> (x != 0?=w15:bool)
              n13 = case shown="True" w15 {
                tunnel: [w18 w24] -> w14
                tunnel: [w18 w23] -> w13
                frame False {
                  n14 = Build Array(0.0) -> (w18:dbl[])
                }
                frame True {
                  n15 = global read "G_VEH.vi" "xobs"() -> (w22:T4)
                  n16 = Unbundle By Name(w22) -> ("x"=w21:dbl, "y"=w20:dbl)
                  n17 = Build Array(w21) -> (w24:dbl[])
                  n18 = Build Array(w20) -> (w23:dbl[])
                }
              }
            }
            frame Disabled {
              w30 = 3 ("disabled index (col)")
              w51 = 3 ("disabled index (col)")
              n19 = global read "G_VEH.vi" "pos_slam"() -> (w38:T2)
              n20 = local read "M6006"() -> (w44:T1)
              n21 = Unbundle By Name(w44) -> ("lcc[1]"=w47:sgl, "lcc[0]"=w46:sgl, "attitude[2]"=w48:sgl)
              n22 = call-poly <vilib>:"A x B.vi"("B"=T2 [[1.0, 0.0, 0.0, 3.0], [0.0, 1.0, 0.0, 0.0], [0.0, 0.0, 1.0, 0.0], [0.0, 0.0, 0.0, 1.0]] ("pos_slam"), "A"=w38) -> ("A x B"=w27:T2)  [unwired: 1 out]
              n23 = local read "M6006"() -> (w35:T1)
              n24 = Unbundle By Name(w35) -> ("lcc[1]"=w32:sgl, "lcc[0]"=w33:sgl, "attitude[2]"=w31:sgl)
              n25 = Index Array(array=w38, index (row) #1=0 ("disabled index (row)"), index (col) #1=w51, index (row) #2=1 ("index (row)"), index (col) #2=w51) -> (element #1=w43:dbl, element #2=w42:dbl)
              n26 = Negate(x=w48) -> (-x=w45:sgl)
              n27 = Index Array(array=w27, index (row) #1=0 ("disabled index (row)"), index (col) #1=w30, index (row) #2=1 ("index (row)"), index (col) #2=w30) -> (element #1=w36:dbl, element #2=w37:dbl)
              n28 = call "rotm_siso.vi"("angle[rad]"=w45, "y0"=w46, "x0"=w47, "y"=w42, "x"=w43) -> ("y'"=w40:dbl, "x'"=w41:dbl)  [unwired: 5 in]
              n29 = Negate(x=w31) -> (-x=w34:sgl)
              n30 = call "rotm_siso.vi"("angle[rad]"=w34, "y0"=w33, "x0"=w32, "y"=w37, "x"=w36) -> ("y'"=w25:dbl, "x'"=w26:dbl)  [unwired: 5 in]
              n31 = Build Array(w41, w26) -> (w50:dbl[])
              n32 = Build Array(w40, w25) -> (w49:dbl[])
            }
          }
          "x 1" <- w12
          "y 1" <- w11
        }
        frame #2 {
          n33 = disable-structure shown="Disabled" {
            disable-tunnel: [w57 _ w77] -> w55
            disable-tunnel: [w56 _ w76] -> w54
            frame Disabled {
              n34 = local read "M6006"() -> (w60:T1)
              n35 = global read "G_VEH.vi" "xyhc_lane"() -> (w68)
              n36 = Unbundle By Name(w60) -> ("lcc[1]"=w64:sgl, "lcc[0]"=w65:sgl, "attitude[2]"=w61:sgl)
              n37 = Unbundle By Name(w68) -> ("x"=w62, "y"=w63)
              n38 = Negate(x=w61) -> (-x=w66:sgl)
              n39 = call "rotm_siso.vi"("angle[rad]"=w66, "reverse"=FALSE, "y0"=w65, "x0"=w64, "y"=w63, "x"=w62) -> ("y'"=w58:dbl, "x'"=w59:dbl)  [unwired: 4 in]
              n40 = Build Array(w59) -> (w57:dbl[])
              n41 = Build Array(w58) -> (w56:dbl[])
            }
            frame Enabled {
            }
            frame Disabled {
              n42 = disable-structure shown="Enabled" {
                disable-tunnel: [w78 w79] -> w75
                frame Enabled {
                  n43 = global read "G_SEN.vi" "Lane_C_M"() -> (w78:dbl[])
                }
                frame Disabled {
                  n44 = global read "G_SEN.vi" "Lane_L_I"() -> (w79:dbl[])
                }
              }
              n45 = Index Array(array=w75, index=0) -> (element=w72:dbl)
              n46 = global read "G_SEN.vi" "M_lane_update"() -> (w70:bool)
              n47 = Greater?(x=w72, y=0.54) -> (0:w69:bool)
              n48 = And(x=w70, y=w69) -> (x .and. y?=w74:bool)
              n49 = case shown="True" w74 {
                tunnel: w75 -> [_ w81]
                tunnel: [_ w82] -> w77
                tunnel: [_ w80] -> w76
                frame False {
                }
                frame True {
                  n50 = global read "G_SEN.vi" "y_mobileye"() -> (w80:dbl[])
                  n51 = Index Array(array=w81, index #1=1 ("index")) -> (element #1=w87:dbl, element #2=w86:dbl, element #3=w83:dbl)  [unwired: 2 in]
                  n52 = Multiply(x=w86, y=w80) -> (x*y=w84:dbl[])
                  n53 = Square(x=w80) -> (x^2=w88:dbl[])
                  n54 = Multiply(x=w87, y=w88) -> (x*y=w85:dbl[])
                  n55 = Compound Arithmetic op=ADD(w85, w84, w83) -> (w82:dbl[])
                }
              }
            }
          }
          "x 2" <- w55
          "y 2" <- w54
        }
        frame #3 {
          n56 = disable-structure shown="Disabled" {
            disable-tunnel: [w93 w108 _] -> w91
            disable-tunnel: [w92 w109 _] -> w90
            frame Disabled {
              n57 = global read "G_VEH.vi" "xlane"() -> (w94:T5)
              n58 = for {
                tunnel: w94 -> [w105] mode=indexing
                tunnel: [w96] -> w93 mode=indexing
                tunnel: [w95] -> w92 mode=indexing
                n59 = Unbundle By Name(w105) -> ("x"=w99:dbl, "y"=w100:dbl)
                n60 = local read "M6006"() -> (w97:T1)
                n61 = Unbundle By Name(w97) -> ("lcc[1]"=w101:sgl, "lcc[0]"=w102:sgl, "attitude[2]"=w98:sgl)
                n62 = Negate(x=w98) -> (-x=w103:sgl)
                n63 = call "rotm_siso.vi"("angle[rad]"=w103, "reverse"=FALSE, "y0"=w102, "x0"=w101, "y"=w100, "x"=w99) -> ("y'"=w95:dbl, "x'"=w96:dbl)  [unwired: 4 in]
              }
            }
            frame Disabled {
              n64 = disable-structure shown="Enabled" {
                disable-tunnel: [w110 w111] -> w107
                frame Enabled {
                  n65 = global read "G_SEN.vi" "Lane_C_M 2"() -> (w110:dbl[])
                }
                frame Disabled {
                  n66 = global read "G_SEN.vi" "Lane_R_I"() -> (w111:dbl[])
                }
              }
              n67 = case shown="True" TRUE {
                tunnel: w107 -> [_ w113]
                tunnel: [_ w114] -> w108
                tunnel: [_ w112] -> w109
                frame False {
                }
                frame True {
                  n68 = global read "G_SEN.vi" "y_mobileye"() -> (w112:dbl[])
                  n69 = Index Array(array=w113, index #1=1 ("index")) -> (element #1=w119:dbl, element #2=w118:dbl, element #3=w115:dbl)  [unwired: 2 in]
                  n70 = Multiply(x=w118, y=w112) -> (x*y=w116:dbl[])
                  n71 = Square(x=w112) -> (x^2=w120:dbl[])
                  n72 = Multiply(x=w119, y=w120) -> (x*y=w117:dbl[])
                  n73 = Compound Arithmetic op=ADD(w117, w116, w115) -> (w114:dbl[])
                }
              }
            }
            frame Enabled {
            }
          }
          "x 3" <- w91
          "y 3" <- w90
        }
        frame #4 {
          n74 = disable-structure shown="Disabled" {
            disable-tunnel: [w129 w177 _ w190 w197] -> w123
            disable-tunnel: [w126 w176 _ w189 w195] -> w122
            frame Disabled {
              n75 = flat-sequence {
                tunnel: [w148] -> w133
                tunnel: [w147] -> w132
                frame #0 {
                  n76 = global read "G_NAV.vi" "M6006"() -> (w164)
                  n77 = Unbundle By Name(w164) -> ("lcc[1]"=w163, "lcc[0]"=w162, "attitude[2]"=w161)
                  n78 = global read "G_SEN.vi" "lane_m"() -> (w159:dbl)
                  n79 = local read "M6006"() -> (w156:T1)
                  n80 = Negate(x=w161) -> (-x=w160:dbl)
                  n81 = Unbundle By Name(w156) -> ("lcc[1]"=w154:sgl, "lcc[0]"=w153:sgl, "attitude[2]"=w155:sgl)
                  n82 = Negate(x=w155) -> (-x=w151:sgl)
                  n83 = call "rotm_siso.vi"("angle[rad]"=w160, "reverse"=TRUE, "y0"=w162, "x0"=w163, "y"=0.0, "x"=w159) -> ("y'"=w149:dbl, "x'"=w150:dbl)  [unwired: 4 in]
                  n84 = call "rotm_siso.vi"("angle[rad]"=w151, "reverse"=FALSE, "y0"=w153, "x0"=w154, "y"=w149, "x"=w150) -> ("y'"=w147:dbl, "x'"=w148:dbl)  [unwired: 4 in]
                }
              }
              n85 = flat-sequence {
                tunnel: [w167] -> w135
                tunnel: [w166] -> w134
                frame #0 {
                  n86 = local read "M6006"() -> (w168:T1)
                  n87 = Unbundle By Name(w168) -> ("lcc[1]"=w172:sgl, "lcc[0]"=w173:sgl, "attitude[2]"=w169:sgl)
                  n88 = global read "G_VEH.vi" "xyhc"() -> (w165)
                  n89 = Unbundle By Name(w165) -> ("x"=w170, "y"=w171)
                  n90 = Negate(x=w169) -> (-x=w174:sgl)
                  n91 = call "rotm_siso.vi"("angle[rad]"=w174, "reverse"=FALSE, "y0"=w173, "x0"=w172, "y"=w171, "x"=w170) -> ("y'"=w166:dbl, "x'"=w167:dbl)  [unwired: 4 in]
                }
              }
              n92 = flat-sequence {
                tunnel: [w138] -> w125
                tunnel: [w137] -> w124
                frame #0 {
                  n93 = local read "M6006"() -> (w139:T1)
                  n94 = Unbundle By Name(w139) -> ("lcc[1]"=w143:sgl, "lcc[0]"=w144:sgl, "attitude[2]"=w140:sgl)
                  n95 = global read "G_VEH.vi" "xtmp"() -> (w136:T4)
                  n96 = Unbundle By Name(w136) -> ("x"=w141:dbl, "y"=w142:dbl)
                  n97 = Negate(x=w140) -> (-x=w145:sgl)
                  n98 = call "rotm_siso.vi"("angle[rad]"=w145, "reverse"=FALSE, "y0"=w144, "x0"=w143, "y"=w142, "x"=w141) -> ("y'"=w137:dbl, "x'"=w138:dbl)  [unwired: 4 in]
                }
              }
              n99 = Build Array(w135, w133, w125, w125) -> (w131:dbl[])
              n100 = Build Array(w134, w132, w124, w124) -> (w127:dbl[])
              n101 = Array Subset(array=w131, length=2) -> (w129:dbl[])  [unwired: 1 in]
              n102 = Array Subset(array=w127, length=2) -> (w126:dbl[])  [unwired: 1 in]
            }
            frame Disabled {
              n103 = local read "M6006"() -> (w180:T1)
              n104 = Unbundle By Name(w180) -> ("lcc[1]"=w184:sgl, "lcc[0]"=w185:sgl, "attitude[2]"=w181:sgl)
              n105 = global read "G_VEH.vi" "xyhc"() -> (w188)
              n106 = Unbundle By Name(w188) -> ("x"=w182, "y"=w183)
              n107 = Negate(x=w181) -> (-x=w186:sgl)
              n108 = call "rotm_siso.vi"("angle[rad]"=w186, "reverse"=FALSE, "y0"=w185, "x0"=w184, "y"=w183, "x"=w182) -> ("y'"=w178:dbl, "x'"=w179:dbl)  [unwired: 4 in]
              n109 = Build Array(w179) -> (w177:dbl[])
              n110 = Build Array(w178) -> (w176:dbl[])
            }
            frame Enabled {
            }
            frame Disabled {
              n111 = global read "G_SEN.vi" "CIPV"() -> (w192:dbl[][])
              n112 = Index Array(array=w192, index (col) #1=1 ("disabled index (col)")) -> (element #1=w190:dbl[], element #2=w189:dbl[])  [unwired: 3 in]
            }
            frame Disabled {
              n113 = flat-sequence {
                tunnel: [w211] -> w198
                tunnel: [w210] -> w196
                frame #0 {
                  n114 = local read "M6006"() -> (w213:T1)
                  n115 = Unbundle By Name(w213) -> ("lcc[1]"=w215:sgl, "lcc[0]"=w216:sgl, "attitude[2]"=w214:sgl)
                  n116 = global read "G_VEH.vi" "xtmp"() -> (w212:T4)
                  n117 = Unbundle By Name(w212) -> ("x"=w211:dbl, "y"=w210:dbl)
                  n118 = Negate(x=w214) -> (-x=w217:sgl)
                  n119 = call "rotm_siso.vi"("angle[rad]"=w217, "reverse"=FALSE, "y0"=w216, "x0"=w215, "y"=w210, "x"=w211) -> ()  [unwired: 4 in, 2 out]
                }
              }
              n120 = flat-sequence {
                tunnel: [w201] -> w194
                tunnel: [w200] -> w193
                frame #0 {
                  n121 = local read "M6006"() -> (w202:T1)
                  n122 = Unbundle By Name(w202) -> ("lcc[1]"=w206:sgl, "lcc[0]"=w207:sgl, "attitude[2]"=w203:sgl)
                  n123 = global read "G_VEH.vi" "xctmp"() -> (w199:T4)
                  n124 = Unbundle By Name(w199) -> ("x"=w204:dbl, "y"=w205:dbl)
                  n125 = Negate(x=w203) -> (-x=w208:sgl)
                  n126 = call "rotm_siso.vi"("angle[rad]"=w208, "reverse"=FALSE, "y0"=w207, "x0"=w206, "y"=w205, "x"=w204) -> ("y'"=w200:dbl, "x'"=w201:dbl)  [unwired: 4 in]
                }
              }
              n127 = Build Array(w198, w194) -> (w197:dbl[])
              n128 = Build Array(w196, w193) -> (w195:dbl[])
            }
          }
          "x 4" <- w123
          "y 4" <- w122
        }
        frame #5 {
          n129 = local read "M6006"() -> (w226:T1)
          n130 = global read "G_NAV.vi" "GPS_status"() -> (w221)
          n131 = Unbundle By Name(w226) -> ("lcc[1]"=w229:sgl, "lcc[0]"=w228:sgl, "attitude[2]"=w230:sgl)
          n132 = Unbundle By Name(w221) -> ("y"=w220, "x"=w219)
          n133 = Negate(x=w230) -> (-x=w227:sgl)
          n134 = call "rotm_siso.vi"("angle[rad]"=w227, "y0"=w228, "x0"=w229, "y"=w219, "x"=w220) -> ("y'"=w223:dbl, "x'"=w225:dbl)  [unwired: 5 in]
          n135 = Build Array(w225) -> (→"x 5":dbl[])
          n136 = Build Array(w223) -> (→"y 5":dbl[])
        }
        frame #6 {
          n137 = disable-structure shown="Disabled" {
            disable-tunnel: [w242 w244 w251 w258 _] -> w232
            disable-tunnel: [w241 w245 w250 w259 _] -> w231
            frame Disabled {
              n138 = local read item#-1() -> (w233)
              n139 = Unbundle By Name(w233) -> ("lcc[1]"=w236, "lcc[0]"=w235, "attitude[2]"=w237)
              n140 = global read "G_SEN.vi" "wpt_park"() -> (w238)
              n141 = Negate(x=w237) -> (-x=w234:dbl)
              n142 = Index Array(array=w238, index (col) #1=0 ("disabled index (col)")) -> (element #1=w239, element #2=w240)  [unwired: 3 in]
              n143 = call "rotm_mimo.vi"("angle[rad]"=w234, "y0"=w235, "x0"=w236, "y"=w240, "x"=w239) -> ("Y"=w242:dbl[], "X"=w241:dbl[])  [unwired: 3 in, 2 out]
            }
            frame Disabled {
              n144 = Index Array(index (col) #1=0 ("disabled index (col)"), index (col) #2=1 ("index (col)")) -> (element #1=w245, element #2=w244)  [unwired: 3 in]
            }
            frame Disabled {
              n145 = global read "G_SEN.vi" "crosswalk"() -> (w252:dbl)
              n146 = Build Array(-5.0 ("element"), 5.0 ("element")) -> (w250:dbl[])
              n147 = Build Array(w252, w252) -> (w251:dbl[])
            }
            frame Disabled {
              n148 = global read "G_NAV.vi" "M6006"() -> (w257)
              n149 = Unbundle By Name(w257) -> ("lcc[1]"=w256, "lcc[0]"=w255)
              n150 = global read "G_VEH.vi" "xwalks"() -> (w254:T5)
              n151 = for {
                tunnel: w254 -> [w275] mode=indexing
                tunnel: w256 -> [w273]
                tunnel: w255 -> [w271]
                tunnel: [w260] -> w253
                tunnel: [w264] -> _
                i -> [w264]
                stop <- w260 stop-if-true
                n152 = Unbundle By Name(w275) -> ("idx"=w263:i32, "x"=w274:dbl, "y"=w272:dbl)
                n153 = Subtract(x=w274, y=w273) -> (x-y=w269:dbl)
                n154 = Subtract(x=w272, y=w271) -> (x-y=w270:dbl)
                n155 = Square(x=w269) -> (x^2=w268:dbl)
                n156 = Square(x=w270) -> (x^2=w267:dbl)
                n157 = Add(x=w268, y=w267) -> (x+y=w266:dbl)
                n158 = Not Equal To 0?(x=w263) -> (x != 0?=w262:bool)
                n159 = Less?(x=w266, y=600.0) -> (x < y?=w261:bool)
                n160 = And(x=w262, y=w261) -> (x .and. y?=w260:bool)
              }
              n161 = case shown="True" w253 {
                tunnel: [_ w292] -> w259
                tunnel: [_ w291] -> w258
                frame False {
                  n162 = global read "G_NAV.vi" "M6006"() -> (w279)
                  n163 = Unbundle By Name(w279) -> ("lcc[1]"=w276, "lcc[0]"=w277, "attitude[2]"=w280)
                  n164 = Negate(x=w280) -> (-x=w278:dbl)
                  n165 = call "rotm_siso.vi"("angle[rad]"=w278, "reverse"=TRUE, "y0"=w277, "x0"=w276, "y"=90.0, "x"=0.0) -> ("y'"=w286:dbl, "x'"=w285:dbl)  [unwired: 4 in]
                  n166 = global read "G_VEH.vi" "xwalk"() -> (w284:T4)
                  n167 = Bundle By Name(cluster=w284, "x"=w285, "y"=w286) -> (w287:T4)
                  n168 = global write "G_VEH.vi" "xwalk"(w287) -> ()
                }
                frame True {
                  n169 = local read "M6006"() -> (w293:T1)
                  n170 = Unbundle By Name(w293) -> ("lcc[1]"=w297:sgl, "lcc[0]"=w298:sgl, "attitude[2]"=w294:sgl)
                  n171 = global read "G_VEH.vi" "xwalk"() -> (w301:T4)
                  n172 = Unbundle By Name(w301) -> ("x"=w295:dbl, "y"=w296:dbl)
                  n173 = Negate(x=w294) -> (-x=w299:sgl)
                  n174 = call "rotm_siso.vi"("angle[rad]"=w299, "reverse"=FALSE, "y0"=w298, "x0"=w297, "y"=w296, "x"=w295) -> ("y'"=w288:dbl)  [unwired: 4 in, 1 out]
                  n175 = Build Array(w288, w288) -> (w291:dbl[])
                  n176 = Build Array(-5.0 ("element"), 5.0 ("element")) -> (w292:dbl[])
                }
              }
            }
            frame Enabled {
            }
          }
          "x 6" <- w231
          "y 6" <- w232
        }
        frame #7 {
          n177 = disable-structure shown="Disabled" {
            disable-tunnel: [w323 w343 w353] -> w318
            frame Enabled {
              n178 = global read "G_VEH.vi" "Rpath"() -> (w323:dbl)
            }
            frame Disabled {
              n179 = global read "G_LCM.vi" "CON_T"() -> (w336:T6)
              n180 = global read "G_VEH.vi" "ratio_steer"() -> (w341:dbl)
              n181 = global read "G_VEH.vi" "ratio_steer"() -> (w347:dbl)
              n182 = Unbundle By Name(w336) -> ("ref_steer"=w335:dbl)
              n183 = global read "G_VEH.vi" "handle"() -> (w345:dbl)
              n184 = Divide(x=w335, y=w341) -> (x/y=w342:dbl)
              n185 = Divide(x=w345, y=w347) -> (x/y=w346:dbl)
              n186 = Multiply(x=w342, y=3.141592653589793) -> (x*y=w338:dbl)
              n187 = Multiply(x=w346, y=3.141592653589793) -> (x*y=w351:dbl)
              n188 = Divide(x=w338, y=180.0) -> (x/y=w340:dbl)
              n189 = Divide(x=w351, y=180.0) -> (x/y=w349:dbl)
              n190 = global read "G_VEH.vi" "C_Wheel base"() -> (w325:dbl)
              n191 = global read "G_VEH.vi" "C_Wheel base"() -> (w348:dbl)
              n192 = Tangent(1:w340) -> (0:w326:dbl)
              n193 = Tangent(1:w349) -> (0:w333:dbl)
              n194 = Divide(x=w325, y=w326) -> (x/y=w328:dbl)
              n195 = Divide(x=w348, y=w333) -> (x/y=w332:dbl)
              n196 = Not Equal To 0?(x=w326) -> (x != 0?=w327:bool)
              n197 = Not Equal To 0?(x=w333) -> (x != 0?=w334:bool)
              n198 = Select(t=w328, s=w327, f=9999999.0) -> (s? t:f=w324:dbl)
              n199 = Select(t=w332, s=w334, f=9999999.0) -> (s? t:f=w331:dbl)
              n200 = local read "replay"() -> (w344:bool)
              n201 = Select(t=w324, s=w344, f=w331) -> (s? t:f=w343:dbl)
            }
            frame Disabled {
              n202 = global read "G_PATH.vi" "RXY"() -> (w358:dbl[])
              n203 = Index Array(array=w358, index #1=0 ("index")) -> (element #1=w354:dbl, element #2=w357:dbl)  [unwired: 1 in]
              n204 = Sign(1:w357) -> (0:w356:dbl)
              n205 = Negate(x=w356) -> (-x=w355:dbl)
              n206 = Multiply(x=w354, y=w355) -> (x*y=w353:dbl)
            }
          }
          n207 = disable-structure shown="Enabled" {
            disable-tunnel: [w320 30.0] -> w304
            frame Disabled {
              n208 = global read "G_VEH.vi" "Preview dist"() -> (w319:dbl)
              n209 = Multiply(x=w319, y=1.5) -> (x*y=w320:dbl)
            }
            frame Enabled {
            }
          }
          n210 = Divide(x=w304, y=w318) -> (x/y=w311:dbl)
          n211 = Equal To 0?(x=w318) -> (x = 0?=w310:bool)
          n212 = Select(t=0.0, s=w310, f=w311) -> (s? t:f=w308:dbl)
          n213 = Absolute Value(x=w308) -> (abs(x)=w309:dbl)
          n214 = Sign(1:w308) -> (0:w306:dbl)
          n215 = call "array_new.vi"("end"=w309, "size"=0.04, "start"=0.0) -> ("Array"=w307:dbl[])  [unwired: 7 in, 1 out]
          n216 = Multiply(x=w307, y=w306) -> (x*y=w305:dbl[])
          n217 = Sine & Cosine(0:w305) -> (1:w313:dbl[], 2:w314:dbl[])
          n218 = Multiply(x=w318, y=w313) -> (x*y=→"y 7":dbl[])
          n219 = Multiply(x=w314, y=w318) -> (x*y=w317:dbl[])
          n220 = Subtract(x=w317, y=w318) -> (x-y=→"x 7":dbl[])
        }
        frame #8 {
          n221 = disable-structure shown="Disabled" {
            disable-tunnel: [w362 _ w383] -> w361
            disable-tunnel: [w363 _ w384] -> w360
            frame Disabled {
              n222 = global read "G_PATH.vi" "map_track_saved"() -> (w370:dbl[][])
              n223 = global read "G_PATH.vi" "map_track"() -> (w371:dbl[][])
              n224 = local read "M6006"() -> (w366:T1)
              n225 = Unbundle By Name(w366) -> ("lcc[1]"=w365:sgl, "lcc[0]"=w364:sgl, "attitude[2]"=w368:sgl)
              n226 = Select(t=w370, s="replay", f=w371) -> (s? t:f=w369:dbl[][])
              n227 = Negate(x=w368) -> (-x=w367:sgl)
              n228 = Index Array(array=w369, index (col) #1=0 ("disabled index (col)"), index (col) #2=1 ("disabled index (col)")) -> (element #1=w363:dbl[], element #2=w362:dbl[])  [unwired: 2 in]
              n229 = call "rotm_mimo.vi"("angle[rad]"=w367, "y0"=w364, "x0"=w365, "y"=w362, "x"=w363) -> ()  [unwired: 3 in, 4 out]
            }
            frame Enabled {
            }
            frame Disabled {
              n230 = global read "G_SEN.vi" "y_mobileye"() -> (w383:dbl[])
              n231 = global read "G_SEN.vi" "Lane_C_M"() -> (w382:dbl[])
              n232 = Square(x=w383) -> (x^2=w380:dbl[])
              n233 = Index Array(array=w382, index #1=1 ("index")) -> (element #1=w379:dbl, element #2=w378:dbl, element #3=w375:dbl)  [unwired: 2 in]
              n234 = Multiply(x=w379, y=w380) -> (x*y=w377:dbl[])
              n235 = Multiply(x=w378, y=w383) -> (x*y=w376:dbl[])
              n236 = Compound Arithmetic op=ADD(w377, w376, w375) -> (w384:dbl[])
            }
          }
          "x 8" <- w360
          "y 8" <- w361
        }
        frame #9 {
          n237 = disable-structure shown="Enabled" {
            disable-tunnel: [w395 w425] -> w386
            disable-tunnel: [w394 w424] -> w385
            frame Enabled {
              n238 = disable-structure shown="Enabled" {
                disable-tunnel: [w403 w417 _] -> w389
                disable-tunnel: [w402 w418 _] -> w388
                frame Disabled {
                  n239 = global read "G_VEH.vi" "xyhc_shift"() -> (w415)
                  n240 = Unbundle By Name(w415) -> ("x"=w401, "y"=w400, "h"=w412)
                  n241 = call "headingoperater.vi"("h1"=w412, "h2"=1.5707963267948966) -> ("h2-h1"=w406:dbl)  [unwired: 8 in, 1 out]
                  n242 = global read "G_VEH.vi" "xyhc_lane"() -> (w404)
                  n243 = Unbundle By Name(w404) -> ("x"=w413, "y"=w414)
                  n244 = Negate(x=w406) -> (-x=w405:dbl)
                  n245 = call "rotm_siso.vi"("angle[rad]"=w405, "y0"=w400, "x0"=w401, "y"=w414, "x"=w413) -> ("x'"=w416:dbl)  [unwired: 5 in, 1 out]
                  n246 = call "rotm_siso.vi"("angle[rad]"=w405, "reverse"=TRUE, "y0"=w400, "x0"=w401, "y"=0.0, "x"=w416) -> ("y'"=w408:dbl, "x'"=w409:dbl)  [unwired: 4 in]
                  n247 = Subtract(x=w409, y=w401) -> (x-y=w402:dbl)
                  n248 = Subtract(x=w408, y=w400) -> (x-y=w403:dbl)
                }
                frame Disabled {
                  n249 = global read "G_PATH.vi" "xt"() -> (w418:dbl)
                  n250 = global read "G_PATH.vi" "yt"() -> (w417:dbl)
                }
                frame Enabled {
                }
              }
              n251 = local read "M6006"() -> (w387:T1)
              n252 = Unbundle By Name(w387) -> ("lcc[1]"=w398:sgl, "lcc[0]"=w397:sgl, "attitude[2]"=w399:sgl)
              n253 = global read "G_PATH.vi" "x origin"() -> (w393:dbl[])
              n254 = global read "G_PATH.vi" "y origin"() -> (w392:dbl[])
              n255 = Add(x=w393, y=w388) -> (x+y=w391:dbl[])
              n256 = Add(x=w392, y=w389) -> (x+y=w390:dbl[])
              n257 = Negate(x=w399) -> (-x=w396:sgl)
              n258 = call "rotm_mimo.vi"("angle[rad]"=w396, "y0"=w397, "x0"=w398, "y"=w390, "x"=w391) -> ("Y"=w394:dbl[], "X"=w395:dbl[])  [unwired: 3 in, 2 out]
            }
            frame Disabled {
              n259 = global read "G_SEN.vi" "Lane_C_I"() -> (w422:dbl[])
              n260 = Index Array(array=w422, index=0) -> (element=w421:dbl)
              n261 = Greater Or Equal?(x=w421, y=0.0) -> (x >= y?=w419:bool)
              n262 = case shown="True" w419 {
                tunnel: w422 -> [_ w430]
                tunnel: [_ w440] -> w425
                tunnel: [_ w428] -> w424
                frame False {
                }
                frame True {
                  n263 = Index Array(array=w430, index=1) -> (element=w427:dbl)
                  n264 = Absolute Value(x=w427) -> (abs(x)=w426:dbl)
                  n265 = Multiply(x=w426, y=2.0) -> (x*y=w437:dbl)
                  n266 = Reciprocal(x=w437) -> (1/x=w436:dbl)
                  n267 = Multiply(x=0.5, y=w436) -> (x*y=w434:dbl)
                  n268 = Round To Nearest(number=w434) -> (nearest integer value=w433:dbl)
                  n269 = Max & Min(x=w433, y=150.0) -> (max(x,y)=w431:dbl)  [unwired: 1 out]
                  n270 = global read "G_SEN.vi" "y_mobileye"() -> (w429:dbl[])
                  n271 = disable-structure shown="Enabled" {
                    disable-tunnel: w431 -> [w450 _]
                    disable-tunnel: w429 -> [w449 w451]
                    disable-tunnel: [w448 w451] -> w428
                    frame Disabled {
                      n272 = Array Subset(array=w449, length=w450) -> (w448:dbl[])  [unwired: 1 in]
                    }
                    frame Enabled {
                    }
                  }
                  n273 = Index Array(array=w430, index #1=1 ("index")) -> (element #1=w445:dbl, element #2=w444:dbl, element #3=w441:dbl)  [unwired: 2 in]
                  n274 = Multiply(x=w444, y=w428) -> (x*y=w442:dbl[])
                  n275 = Square(x=w428) -> (x^2=w446:dbl[])
                  n276 = Multiply(x=w445, y=w446) -> (x*y=w443:dbl[])
                  n277 = Compound Arithmetic op=ADD(w443, w442, w441) -> (w440:dbl[])
                }
              }
            }
          }
          "x 9" <- w386
          "y 9" <- w385
        }
        frame #10 {
          n278 = disable-structure shown="Disabled" {
            disable-tunnel: [w460 _] -> w453
            disable-tunnel: [w459 _] -> w452
            frame Disabled {
              n279 = global read "G_SEN.vi" "Lane_L_M"() -> (w457:dbl[])
              n280 = Index Array(array=w457, index=0) -> (element=w455:dbl)
              n281 = Greater?(x=w455, y=0.65) -> (0:w456:bool)
              n282 = case shown="True" w456 {
                tunnel: w457 -> [_ w462]
                tunnel: [_ w463] -> w460
                tunnel: [_ w461] -> w459
                frame False {
                }
                frame True {
                  n283 = global read "G_SEN.vi" "y_mobileye"() -> (w461:dbl[])
                  n284 = Index Array(array=w462, index #1=1 ("index")) -> (element #1=w468:dbl, element #2=w467:dbl, element #3=w464:dbl)  [unwired: 2 in]
                  n285 = Multiply(x=w467, y=w461) -> (x*y=w465:dbl[])
                  n286 = Square(x=w461) -> (x^2=w469:dbl[])
                  n287 = Multiply(x=w468, y=w469) -> (x*y=w466:dbl[])
                  n288 = Compound Arithmetic op=ADD(w466, w465, w464) -> (w463:dbl[])
                }
              }
            }
            frame Enabled {
            }
          }
          "x 10" <- w453
          "y 10" <- w452
        }
        frame #11 {
          n289 = disable-structure shown="Disabled" {
            disable-tunnel: [w479 _] -> w472
            disable-tunnel: [w478 _] -> w471
            frame Disabled {
              n290 = global read "G_SEN.vi" "Lane_R_M"() -> (w476:dbl[])
              n291 = Index Array(array=w476, index=0) -> (element=w474:dbl)
              n292 = Greater?(x=w474, y=0.65) -> (0:w475:bool)
              n293 = case shown="True" w475 {
                tunnel: w476 -> [_ w481]
                tunnel: [_ w482] -> w479
                tunnel: [_ w480] -> w478
                frame False {
                }
                frame True {
                  n294 = global read "G_SEN.vi" "y_mobileye"() -> (w480:dbl[])
                  n295 = Index Array(array=w481, index #1=1 ("index")) -> (element #1=w487:dbl, element #2=w486:dbl, element #3=w483:dbl)  [unwired: 2 in]
                  n296 = Multiply(x=w486, y=w480) -> (x*y=w484:dbl[])
                  n297 = Square(x=w480) -> (x^2=w488:dbl[])
                  n298 = Multiply(x=w487, y=w488) -> (x*y=w485:dbl[])
                  n299 = Compound Arithmetic op=ADD(w485, w484, w483) -> (w482:dbl[])
                }
              }
            }
            frame Enabled {
            }
          }
          "x 11" <- w472
          "y 11" <- w471
        }
        frame #12 {
          n300 = disable-structure shown="Enabled" {
            disable-tunnel: [w496 w499 _] -> w491
            disable-tunnel: [w495 w500 _] -> w490
            frame Disabled {
              n301 = disable-structure shown="Disabled" {
                disable-tunnel: [w497 w498 _] -> w494
                frame Disabled {
                  n302 = global read "G_SEN.vi" "sensor_etc"() -> (w497:dbl[][])
                }
                frame Enabled {
                  n303 = global read "G_SEN.vi" "sensor_temp"() -> (w498)
                }
                frame Disabled {
                  n304 = global read "G_SEN.vi" "sensor_obs_log"() -> ()  [unwired: 1 out]
                }
              }
              n305 = Index Array(array=w494, index (col) #1=0 ("disabled index (col)"), index (col) #2=1 ("index (col)")) -> (element #1=w495:dbl[], element #2=w496:dbl[])  [unwired: 2 in]
            }
            frame Disabled {
              n306 = global read "G_NAV.vi" "M6006"() -> (w503)
              n307 = global read "G_SEN.vi" "sensor_obs_log"() -> (w508:dbl[][])
              n308 = Unbundle By Name(w503) -> ("lcc[1]"=w507, "lcc[0]"=w506, "attitude[2]"=w505)
              n309 = Negate(x=w505) -> (-x=w504:dbl)
              n310 = Index Array(array=w508, index (col) #1=0 ("disabled index (col)")) -> (element #1=w502:dbl[], element #2=w501:dbl[])  [unwired: 3 in]
              n311 = call "rotm_mimo.vi"("angle[rad]"=w504, "y0"=w506, "x0"=w507, "y"=w501, "x"=w502) -> ("Y"=w499:dbl[], "X"=w500:dbl[])  [unwired: 3 in, 2 out]
            }
            frame Enabled {
            }
          }
          "x 12" <- w490
          "y 12" <- w491
        }
        frame #13 {
          n312 = disable-structure shown="Enabled" {
            disable-tunnel: [w513 _] -> w511
            disable-tunnel: [w512 _] -> w510
            frame Disabled {
              n313 = flat-sequence {
                tunnel: [w515] -> w513
                tunnel: [w514] -> w512
                frame #0 {
                  n314 = global read "G_SEN.vi" "sensor_obs"() -> (w518:dbl[][])
                  n315 = Index Array(array=w518, index (col) #1=0 ("disabled index (col)"), index (col) #2=1 ("index (col)")) -> (element #1=w517:dbl[], element #2=w516:dbl[])  [unwired: 2 in]
                  n316 = disable-structure shown="Enabled" {
                    disable-tunnel: w517 -> [w537 w539]
                    disable-tunnel: w516 -> [w536 w538]
                    disable-tunnel: [w522 w539] -> w515
                    disable-tunnel: [w521 w538] -> w514
                    frame Disabled {
                      n317 = global read "G_VEH.vi" "xsensor"() -> (w533:T4)
                      n318 = local read "M6006"() -> (w527:T1)
                      n319 = Unbundle By Name(w533) -> ("x"=w535:dbl, "y"=w534:dbl, "h"=w532:dbl)
                      n320 = Unbundle By Name(w527) -> ("lcc[1]"=w526:sgl, "lcc[0]"=w525:sgl, "attitude[2]"=w524:sgl)
                      n321 = Negate(x=w532) -> (-x=w531:dbl)
                      n322 = Negate(x=w524) -> (-x=w523:sgl)
                      n323 = call "rotm_mimo.vi"("angle[rad]"=w531, "reverse"=TRUE, "y0"=w534, "x0"=w535, "y"=w536, "x"=w537) -> ("Y"=w528:dbl[], "X"=w529:dbl[])  [unwired: 2 in, 2 out]
                      n324 = call "rotm_mimo.vi"("angle[rad]"=w523, "y0"=w525, "x0"=w526, "y"=w528, "x"=w529) -> ("Y"=w521:dbl[], "X"=w522:dbl[])  [unwired: 3 in, 2 out]
                    }
                    frame Enabled {
                    }
                  }
                }
              }
            }
            frame Enabled {
            }
          }
          "x 13" <- w511
          "y 13" <- w510
        }
        frame #14 {
          n325 = disable-structure shown="Disabled" {
            disable-tunnel: [w543 _] -> w541
            disable-tunnel: [w542 _] -> w540
            frame Disabled {
              n326 = disable-structure shown="Enabled" {
                disable-tunnel: [w544 w549 w565] -> w542
                disable-tunnel: [w545 w548 w564] -> w543
                frame Disabled {
                  n327 = global read "G_SEN.vi" "sensor_lane"() -> (w546:dbl[][])
                  n328 = Index Array(array=w546, index (col) #1=0 ("disabled index (col)")) -> (element #1=w545:dbl[], element #2=w544:dbl[])  [unwired: 3 in]
                }
                frame Enabled {
                  n329 = global read "G_NAV.vi" "M6006"() -> (w552)
                  n330 = global read "G_SEN.vi" "sensor_lane_log"() -> (w557:dbl[][])
                  n331 = Unbundle By Name(w552) -> ("lcc[1]"=w556, "lcc[0]"=w555, "attitude[2]"=w554)
                  n332 = Negate(x=w554) -> (-x=w553:dbl)
                  n333 = Index Array(array=w557, index (col) #1=0 ("disabled index (col)")) -> (element #1=w551:dbl[], element #2=w550:dbl[])  [unwired: 3 in]
                  n334 = call "rotm_mimo.vi"("angle[rad]"=w553, "y0"=w555, "x0"=w556, "y"=w550, "x"=w551) -> ("Y"=w549:dbl[], "X"=w548:dbl[])  [unwired: 3 in, 2 out]
                }
                frame Disabled {
                  n335 = global read "G_SEN.vi" "lane_log_RR"() -> (w559:dbl[][])
                  n336 = global read "G_SEN.vi" "lane_log_LL"() -> (w560:dbl[][])
                  n337 = global read "G_SEN.vi" "lane_log_L"() -> (w563:dbl[][])
                  n338 = global read "G_SEN.vi" "lane_log_R"() -> (w562:dbl[][])
                  n339 = global read "G_NAV.vi" "M6006"() -> (w568)
                  n340 = Unbundle By Name(w568) -> ("lcc[1]"=w572, "lcc[0]"=w571, "attitude[2]"=w570)
                  n341 = Build Array (concatenate)(w560, w563, w562, w559) -> (w561:dbl[][])
                  n342 = Negate(x=w570) -> (-x=w569:dbl)
                  n343 = Index Array(array=w561, index (col) #1=0 ("disabled index (col)")) -> (element #1=w567:dbl[], element #2=w566:dbl[])  [unwired: 3 in]
                  n344 = call "rotm_mimo.vi"("angle[rad]"=w569, "y0"=w571, "x0"=w572, "y"=w566, "x"=w567) -> ("Y"=w565:dbl[], "X"=w564:dbl[])  [unwired: 3 in, 2 out]
                }
              }
            }
            frame Enabled {
            }
          }
          "x 14" <- w541
          "y 14" <- w540
        }
        frame #15 {
          n345 = disable-structure shown="Disabled" {
            disable-tunnel: [w577 _] -> w575
            disable-tunnel: [w576 _] -> w574
            frame Disabled {
              n346 = flat-sequence {
                tunnel: [w579] -> w577
                tunnel: [w578] -> w576
                frame #0 {
                  n347 = global read "G_VEH.vi" "xsensor"() -> (w590:T4)
                  n348 = global read "G_SEN.vi" "sensor_lane"() -> (w595:dbl[][])
                  n349 = local read "M6006"() -> (w584:T1)
                  n350 = Unbundle By Name(w590) -> ("x"=w592:dbl, "y"=w591:dbl, "h"=w589:dbl)
                  n351 = Unbundle By Name(w584) -> ("lcc[1]"=w583:sgl, "lcc[0]"=w582:sgl, "attitude[2]"=w581:sgl)
                  n352 = Negate(x=w589) -> (-x=w588:dbl)
                  n353 = Index Array(array=w595, index (col) #1=0 ("disabled index (col)"), index (col) #2=1 ("index (col)")) -> (element #1=w594:dbl[], element #2=w593:dbl[])  [unwired: 2 in]
                  n354 = Negate(x=w581) -> (-x=w580:sgl)
                  n355 = call "rotm_mimo.vi"("angle[rad]"=w588, "reverse"=TRUE, "y0"=w591, "x0"=w592, "y"=w593, "x"=w594) -> ("Y"=w585:dbl[], "X"=w586:dbl[])  [unwired: 2 in, 2 out]
                  n356 = call "rotm_mimo.vi"("angle[rad]"=w580, "y0"=w582, "x0"=w583, "y"=w585, "x"=w586) -> ("Y"=w578:dbl[], "X"=w579:dbl[])  [unwired: 3 in, 2 out]
                }
              }
            }
            frame Enabled {
            }
          }
          "x 15" <- w575
          "y 15" <- w574
        }
        frame #16 {
          n357 = disable-structure shown="Disabled" {
            disable-tunnel: [dbl[] [-0.925, -0.925, -0.925, -0.6775, -0.6775, -0.925, -0.925, -0.925, -0.925, -0.6775, -0.6775, -0.925, -0.925, -0.925, 0.9025, 0.9025, 0.9025, 0.6775, 0.6775, 0.9025, 0.9025, 0.9025, 0.9025, 0.6775, 0.6775, 0.9025, 0.9025, 0.9025, -0.925] ("car_x") _] -> w599
            disable-tunnel: [dbl[] [-0.75, -0.224, 0.224, 0.224, -0.224, -0.224, 0.224, 2.415, 2.885, 2.885, 2.415, 2.415, 2.885, 3.5, 3.5, 2.885, 2.415, 2.415, 2.885, 2.885, 2.415, 0.224, -0.224, -0.224, 0.224, 0.224, -0.224, -0.75, -0.75] ("car_y") _] -> w598
            frame Disabled {
            }
            frame Enabled {
            }
          }
          "x 16" <- w599
          "y 16" <- w598
        }
        frame #17 {
          n358 = disable-structure shown="Enabled" {
            disable-tunnel: [w607 w608] -> w605
            disable-tunnel: [1 ("disabled index (col)") _] -> w604
            frame Disabled {
              n359 = global read "G_SEN.vi" "sensor_velodyne"() -> (w607)
            }
            frame Enabled {
              n360 = disable-structure shown="Disabled" {
                disable-tunnel: [w609 _] -> w608
                frame Disabled {
                  n361 = global read "G_SEN.vi" "sensor_velodyne_chopped"() -> (w609:dbl[][])
                }
                frame Enabled {
                }
              }
            }
          }
          n362 = Index Array(array=w605, index (col) #1=w604) -> (element #1=→"x 17":dbl[], element #2=→"y 17":dbl[])  [unwired: 3 in]
        }
      }
    }
    frame #1 {
      n363 = flat-sequence {
        tunnel: [w645] -> w611
        frame #0 {
          n364 = local read "x 10"() -> (w637:dbl[])
          n365 = local read "x 11"() -> (w633:dbl[])
          n366 = local read "x 12"() -> (w631:dbl[])
          n367 = local read "x 13"() -> (w629:dbl[])
          n368 = local read "x 14"() -> (w626:dbl[])
          n369 = local read "x 15"() -> (w628:dbl[])
          n370 = local read "x 16"() -> (w615:dbl[])
          n371 = local read "x 17"() -> (w614:dbl[])
          n372 = local read "x 1"() -> (w647:dbl[])
          n373 = local read "x 2"() -> (w644:dbl[])
          n374 = local read "x 3"() -> (w642:dbl[])
          n375 = local read "x 4"() -> (w619:dbl[])
          n376 = local read "x 5"() -> (w617:dbl[])
          n377 = local read "x 6"() -> (w640:dbl[])
          n378 = local read "x 7"() -> (w639:dbl[])
          n379 = local read "x 8"() -> (w634:dbl[])
          n380 = local read "x 9"() -> (w636:dbl[])
          n381 = call "Convert to Dynamic Data9"("Array"=w637) -> ("Dynamic Data Type"=w625:dynamicdata)  [unwired: 3 in]
          n382 = call "Convert to Dynamic Data17"("Array"=w633) -> ("Dynamic Data Type"=w632:dynamicdata)  [unwired: 3 in]
          n383 = call "Convert to Dynamic Data18"("Array"=w631) -> ("Dynamic Data Type"=w630:dynamicdata)  [unwired: 3 in]
          n384 = call "Convert to Dynamic Data21"("Array"=w629) -> ("Dynamic Data Type"=w627:dynamicdata)  [unwired: 3 in]
          n385 = call "Convert to Dynamic Data26"("Array"=w626) -> ("Dynamic Data Type"=w620:dynamicdata)  [unwired: 3 in]
          n386 = call "Convert to Dynamic Data22"("Array"=w628) -> ("Dynamic Data Type"=w621:dynamicdata)  [unwired: 3 in]
          n387 = call "Convert to Dynamic Data24"("Array"=w615) -> ("Dynamic Data Type"=w622:dynamicdata)  [unwired: 3 in]
          n388 = call "Convert to Dynamic Data34"("Array"=w614) -> ("Dynamic Data Type"=w613:dynamicdata)  [unwired: 3 in]
          n389 = call "Convert to Dynamic Data"("Array"=w647) -> ("Dynamic Data Type"=w646:dynamicdata)  [unwired: 3 in]
          n390 = call "Convert to Dynamic Data3"("Array"=w644) -> ("Dynamic Data Type"=w643:dynamicdata)  [unwired: 3 in]
          n391 = call "Convert to Dynamic Data5"("Array"=w642) -> ("Dynamic Data Type"=w641:dynamicdata)  [unwired: 3 in]
          n392 = call "Convert to Dynamic Data29"("Array"=w619) -> ("Dynamic Data Type"=w618:dynamicdata)  [unwired: 3 in]
          n393 = call "Convert to Dynamic Data31"("Array"=w617) -> ("Dynamic Data Type"=w616:dynamicdata)  [unwired: 3 in]
          n394 = call "Convert to Dynamic Data27"("Array"=w640) -> ("Dynamic Data Type"=w623:dynamicdata)  [unwired: 3 in]
          n395 = call "Convert to Dynamic Data7"("Array"=w639) -> ("Dynamic Data Type"=w638:dynamicdata)  [unwired: 3 in]
          n396 = call "Convert to Dynamic Data14"("Array"=w634) -> ("Dynamic Data Type"=w624:dynamicdata)  [unwired: 3 in]
          n397 = call "Convert to Dynamic Data11"("Array"=w636) -> ("Dynamic Data Type"=w635:dynamicdata)  [unwired: 3 in]
          n398 = Merge Signals(w646, w643, w641, w618, w616, w623, w638, w624, w635, w625, w632, w630, w627, w620, w621, w622, w613) -> (w645:dynamicdata)
        }
      }
      n399 = flat-sequence {
        tunnel: [w680] -> w610
        frame #0 {
          n400 = local read "y 10"() -> (w672:dbl[])
          n401 = local read "y 11"() -> (w668:dbl[])
          n402 = local read "y 12"() -> (w666:dbl[])
          n403 = local read "y 13"() -> (w664:dbl[])
          n404 = local read "y 14"() -> (w661:dbl[])
          n405 = local read "y 15"() -> (w662:dbl[])
          n406 = local read "y 16"() -> (w650:dbl[])
          n407 = local read "y 17"() -> (w649:dbl[])
          n408 = local read "y 1"() -> (w682:dbl[])
          n409 = local read "y 2"() -> (w679:dbl[])
          n410 = local read "y 3"() -> (w677:dbl[])
          n411 = local read "y 4"() -> (w654:dbl[])
          n412 = local read "y 5"() -> (w652:dbl[])
          n413 = local read "y 6"() -> (w675:dbl[])
          n414 = local read "y 7"() -> (w674:dbl[])
          n415 = local read "y 8"() -> (w669:dbl[])
          n416 = local read "y 9"() -> (w671:dbl[])
          n417 = call "Convert to Dynamic Data10"("Array"=w672) -> ("Dynamic Data Type"=w660:dynamicdata)  [unwired: 3 in]
          n418 = call "Convert to Dynamic Data15"("Array"=w668) -> ("Dynamic Data Type"=w667:dynamicdata)  [unwired: 3 in]
          n419 = call "Convert to Dynamic Data16"("Array"=w666) -> ("Dynamic Data Type"=w665:dynamicdata)  [unwired: 3 in]
          n420 = call "Convert to Dynamic Data19"("Array"=w664) -> ("Dynamic Data Type"=w663:dynamicdata)  [unwired: 3 in]
          n421 = call "Convert to Dynamic Data25"("Array"=w661) -> ("Dynamic Data Type"=w655:dynamicdata)  [unwired: 3 in]
          n422 = call "Convert to Dynamic Data20"("Array"=w662) -> ("Dynamic Data Type"=w656:dynamicdata)  [unwired: 3 in]
          n423 = call "Convert to Dynamic Data23"("Array"=w650) -> ("Dynamic Data Type"=w657:dynamicdata)  [unwired: 3 in]
          n424 = call "Convert to Dynamic Data33"("Array"=w649) -> ("Dynamic Data Type"=w648:dynamicdata)  [unwired: 3 in]
          n425 = call "Convert to Dynamic Data2"("Array"=w682) -> ("Dynamic Data Type"=w681:dynamicdata)  [unwired: 3 in]
          n426 = call "Convert to Dynamic Data4"("Array"=w679) -> ("Dynamic Data Type"=w678:dynamicdata)  [unwired: 3 in]
          n427 = call "Convert to Dynamic Data6"("Array"=w677) -> ("Dynamic Data Type"=w676:dynamicdata)  [unwired: 3 in]
          n428 = call "Convert to Dynamic Data30"("Array"=w654) -> ("Dynamic Data Type"=w653:dynamicdata)  [unwired: 3 in]
          n429 = call "Convert to Dynamic Data32"("Array"=w652) -> ("Dynamic Data Type"=w651:dynamicdata)  [unwired: 3 in]
          n430 = call "Convert to Dynamic Data28"("Array"=w675) -> ("Dynamic Data Type"=w658:dynamicdata)  [unwired: 3 in]
          n431 = call "Convert to Dynamic Data8"("Array"=w674) -> ("Dynamic Data Type"=w673:dynamicdata)  [unwired: 3 in]
          n432 = call "Convert to Dynamic Data13"("Array"=w669) -> ("Dynamic Data Type"=w659:dynamicdata)  [unwired: 3 in]
          n433 = call "Convert to Dynamic Data12"("Array"=w671) -> ("Dynamic Data Type"=w670:dynamicdata)  [unwired: 3 in]
          n434 = Merge Signals(w681, w678, w676, w653, w651, w658, w673, w659, w670, w660, w667, w665, w663, w655, w656, w657, w648) -> (w680:dynamicdata)
        }
      }
      n435 = call "GRAPH"("Y Input"=w610, "X Input"=w611) -> ("XY Graph"=→"XY Graph":cluster{"Y":dbl[], "Y":dbl[]}[])  [unwired: 3 in, 6 out]
    }
  }
